vi "Parser.vi"(2 "error IO":errorcluster, 3 "ParserStateIN":T1) -> (0 "error out":errorcluster, 1 "ParserStateOUT":T1)   [LabVIEW 2010]
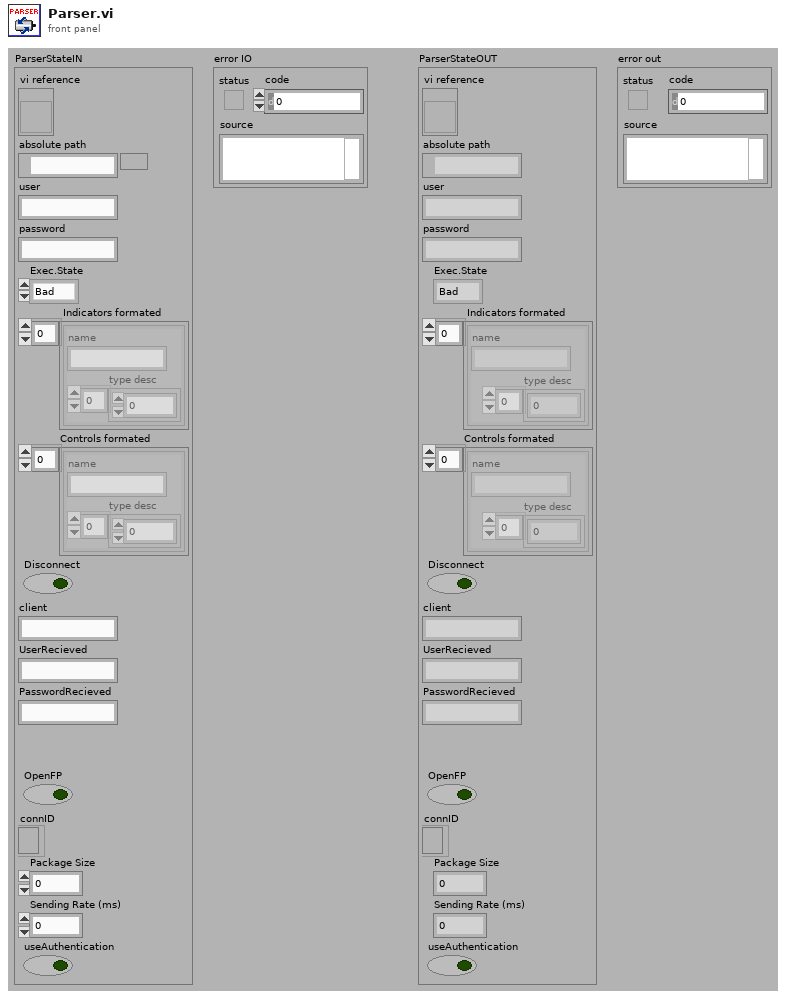
[diagram p1: front panel]
types:
  T1 = cluster{"vi reference":refnum<vi>, "absolute path":path, "user":string, "password":string, "Exec.State":enum32{"Bad", "Idle", "Run top level", "Running"}, " Indicators formated":cluster{"name":string, "type desc":i16[]}[], "Controls formated":cluster{"name":string, "type desc":i16[]}[], "Disconnect":bool, "client":string, "UserRecieved":string, "PasswordRecieved":string, "OpenFP":bool, "connID":refnum<k5>, "Package Size":u32, "Sending Rate (ms)":u32, "useAuthentication":bool}
  T2 = enum32{"Bad", "Idle", "Run top level", "Running"}
  T3 = enum16{"open", "replace", "create", "open or create", "replace or create", "replace or create with confirmation"}
  T4 = typedef "imagedata.ctl" = cluster{"image type":i32, "image depth":i32, "image":u8[], "mask":u8[], "colors":u32[], "Rectangle":cluster{"left":i16, "top":i16, "right":i16, "bottom":i16}}
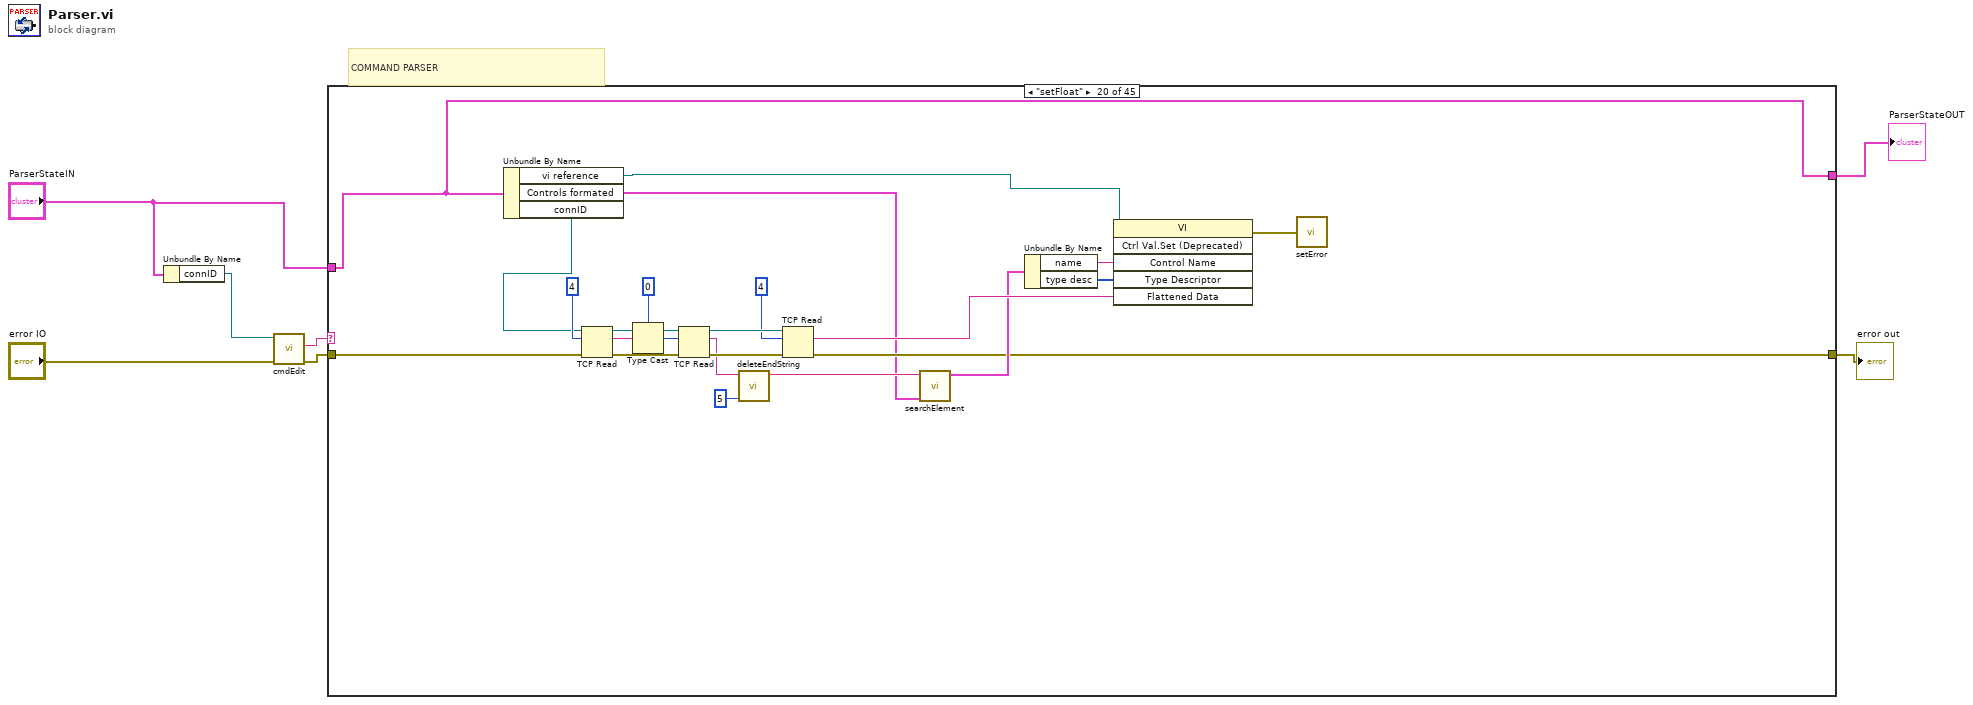
[diagram p0: block diagram]
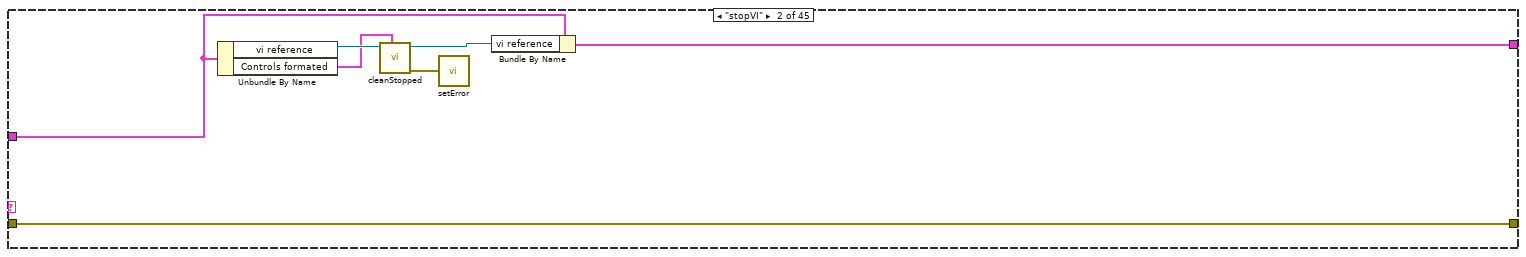
[diagram p3: hidden frame]
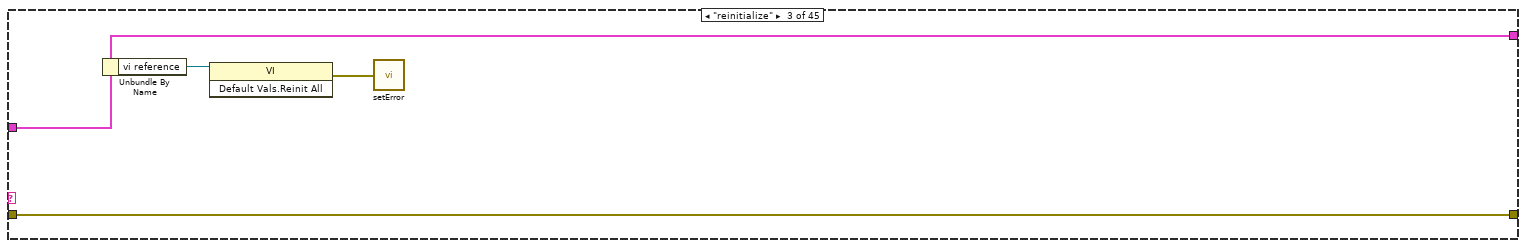
[diagram p4: hidden frame]
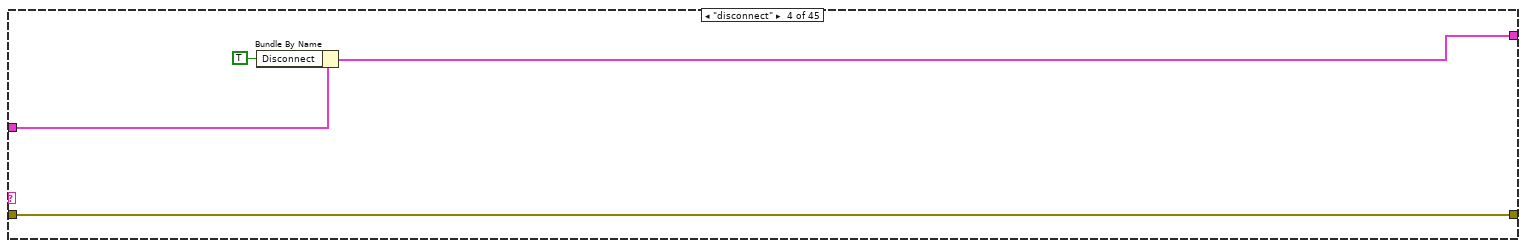
[diagram p5: hidden frame]
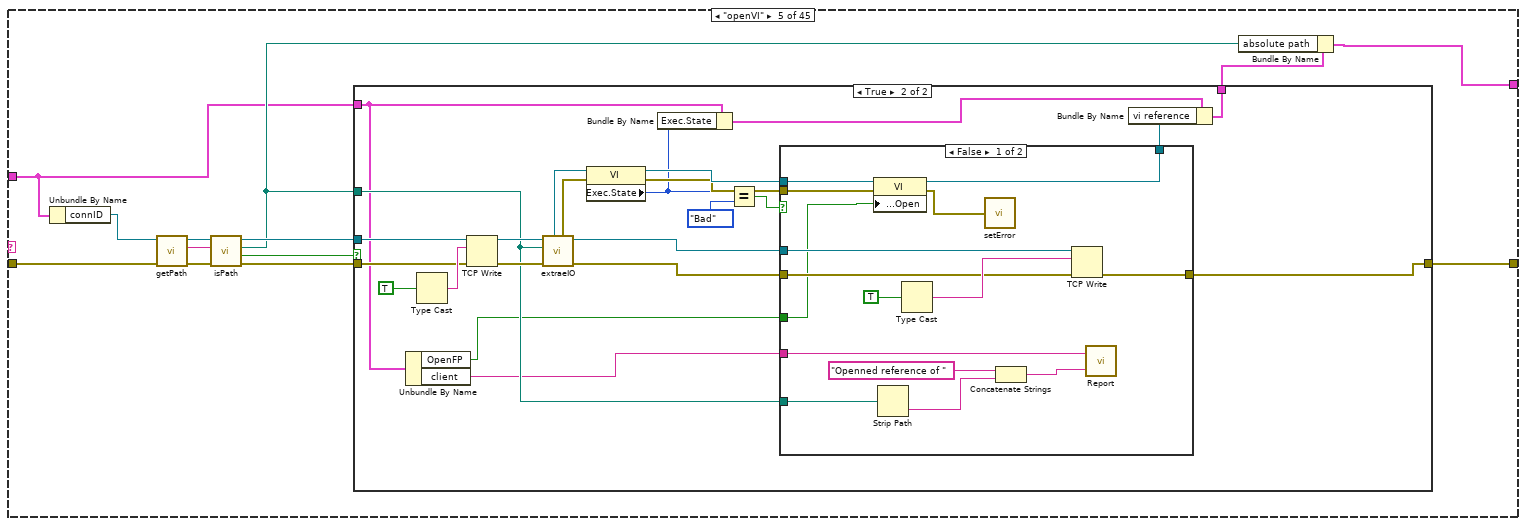
[diagram p6: hidden frame]
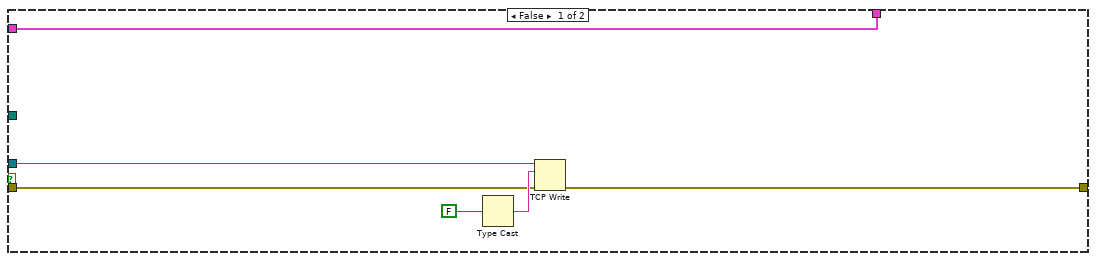
[diagram p7: hidden frame]
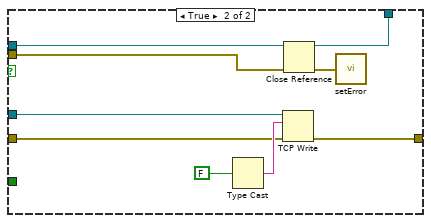
[diagram p8: hidden frame]
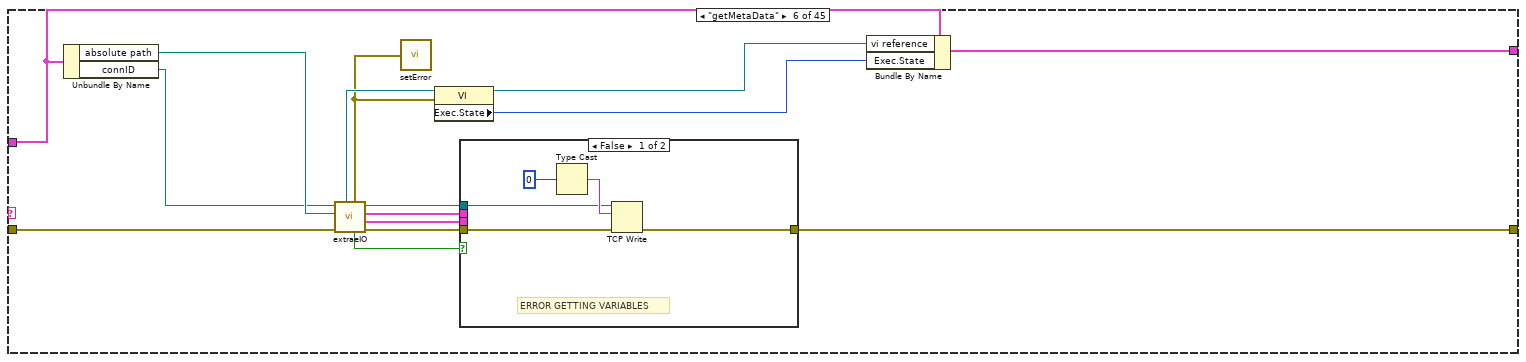
[diagram p9: hidden frame]
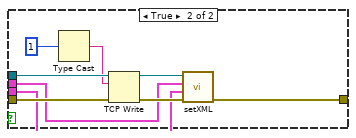
[diagram p10: hidden frame]
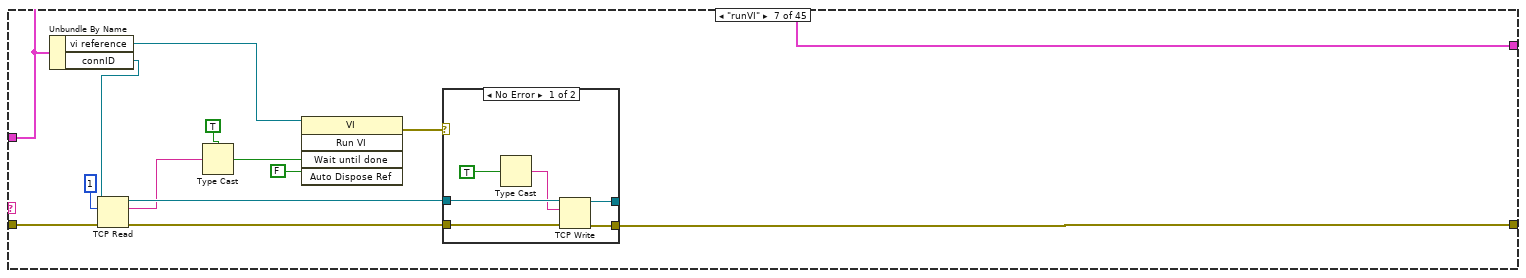
[diagram p11: hidden frame]
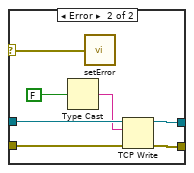
[diagram p12: hidden frame]
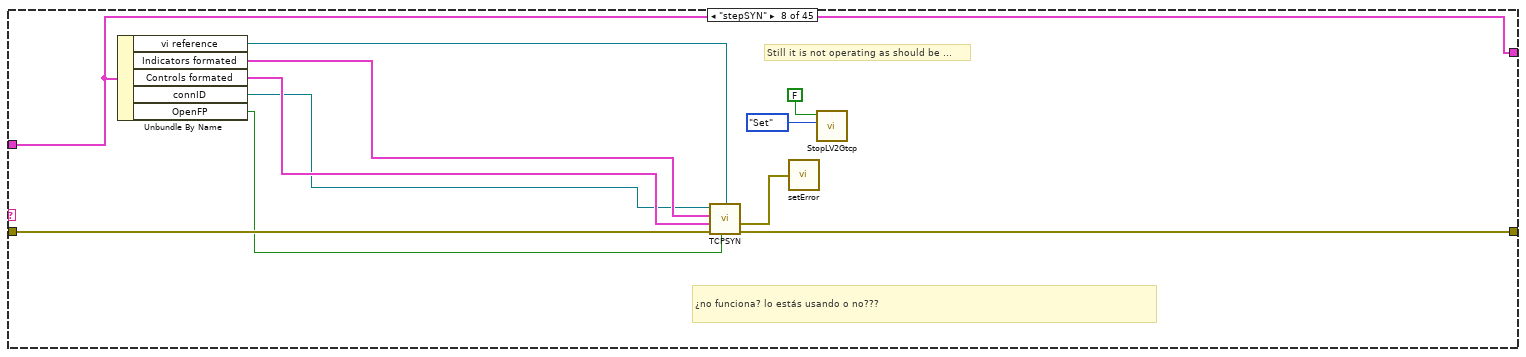
[diagram p13: hidden frame]
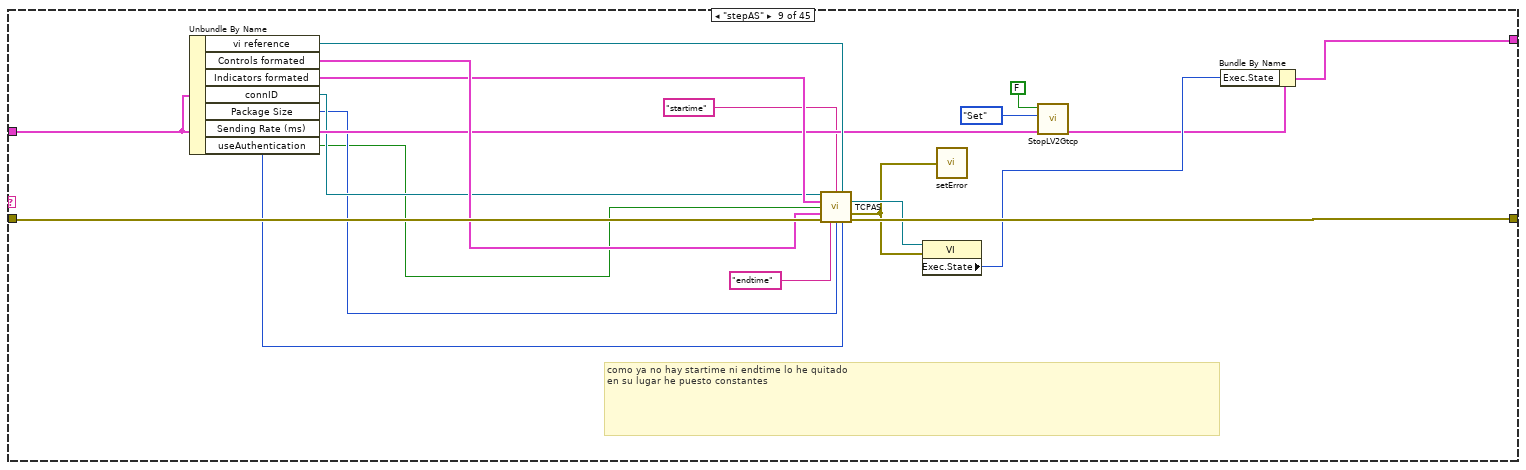
[diagram p14: hidden frame]
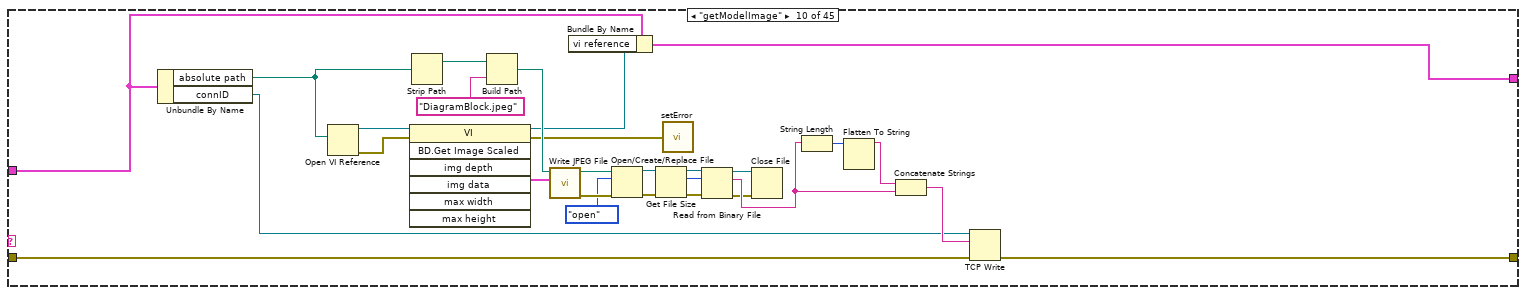
[diagram p15: hidden frame]
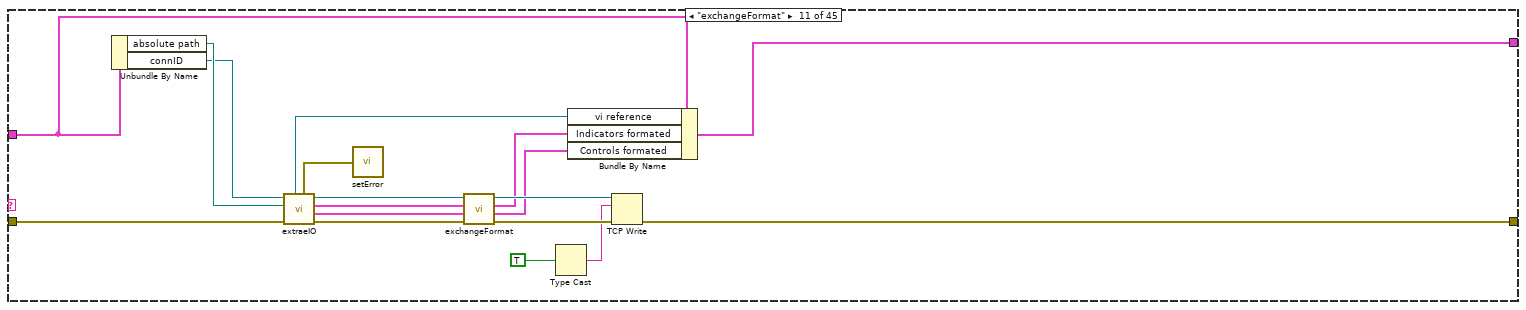
[diagram p16: hidden frame]
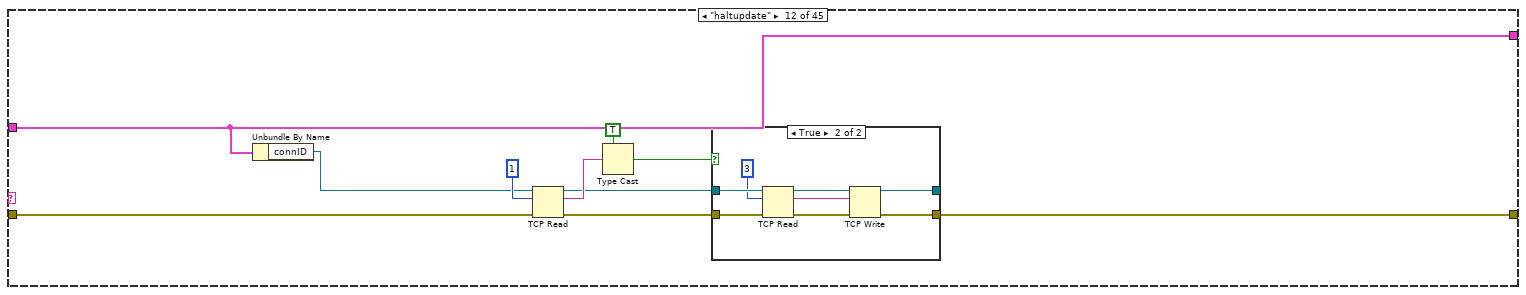
[diagram p17: hidden frame]
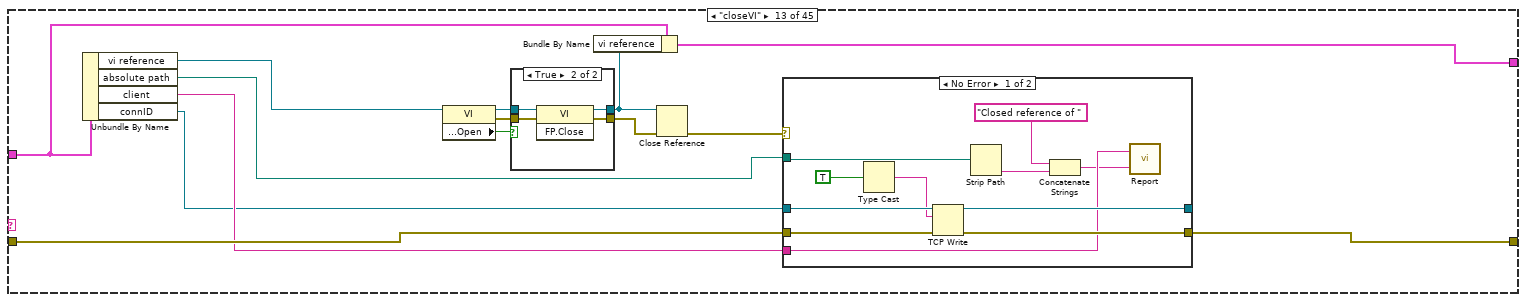
[diagram p19: hidden frame]
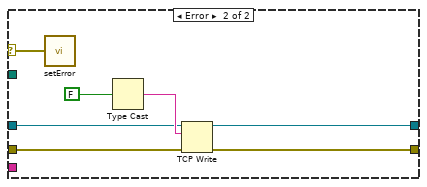
[diagram p20: hidden frame]
diagram:
  # "COMMAND PARSER"
  n1 = Unbundle By Name("ParserStateIN") -> ("connID"=w7:refnum<k5>)
  n2 = call "cmdEdit.vi"("error in (no error)"="error IO", "connection ID"=w7) -> ("error out"=w2:errorcluster, "Command"=w3:string)  [unwired: 8 out]
  n3 = case shown="\"setFloat\"" w3 {
    tunnel: w2 -> [w9 w16 w20 w24 w34 w100 w131 w155 w171 w197 w219 w229 w248 w296 w319 w326 w350 w372 w395 w424 w447 w478 w512 w549 w583 w618 w656 w694 w736 w780 w823 w841 w862 w883 w903 w925 w946 w967 w988 w1008 w1030 w1051 w1072 w1091 w1113]
    tunnel: [w9 w16 w20 w24 w30 w104 w129 w154 w170 w201 w212 w222 w247 w285 w319 w325 w349 w371 w394 w423 w446 w479 w511 w545 w584 w617 w655 w693 w731 w779 w819 w840 w861 w882 w902 w924 w945 w966 w987 w1007 w1029 w1050 w1071 w1092 w1112] -> w4
    tunnel: "ParserStateIN" -> [w8 w15 w17 w23 w26 w91 w120 w147 w163 w177 w206 w221 w245 w281 w318 w321 w344 w367 w390 w419 w442 w475 w508 w541 w580 w613 w651 w689 w727 w776 w816 w835 w856 w877 w900 w919 w942 w962 w982 w1003 w1026 w1045 w1066 w1087 w1109]
    tunnel: [w8 w10 w17 w21 w27 w92 w120 w147 w162 w175 w203 w221 w243 w284 w318 w321 w344 w367 w390 w419 w442 w475 w508 w541 w580 w613 w651 w689 w727 w776 w816 w835 w856 w877 w900 w919 w942 w962 w982 w1003 w1026 w1045 w1066 w1087 w1109] -> w5
    frame "", Default {
    }
    frame "stopVI" {
      n4 = Unbundle By Name(w15) -> ("vi reference"=w13:refnum<vi>, "Controls formated"=w11:cluster{"name":string, "type desc":i16[]}[])
      n5 = call "cleanStopped.vi"("input Controls"=w11, "vi reference in"=w13) -> ("error out"=w12:errorcluster, "vi reference out"=w14:refnum<vi>)  [unwired: 1 in, 7 out]
      n6 = call "setError.vi"("error"=w12) -> ()  [unwired: 1 out]
      n7 = Bundle By Name(cluster=w15, "vi reference"=w14) -> (w10:T1)
    }
    frame "reinitialize" {
      n8 = Unbundle By Name(w17) -> ("vi reference"=w18:refnum<vi>)
      n9 = invoke class="VI" method="Default Vals.Reinit All"(reference=w18) -> (error out=w19:errorcluster)  [unwired: 2 in, 2 out]
      n10 = call "setError.vi"("error"=w19) -> ()  [unwired: 1 out]
    }
    frame "disconnect" {
      n11 = Bundle By Name(cluster=w23, "Disconnect"=TRUE) -> (w21:T1)
    }
    frame "openVI" {
      n12 = Unbundle By Name(w26) -> ("connID"=w25:refnum<k5>)
      n13 = call "getPath.vi"("error in TCP"=w34, "connection ID in"=w25) -> ("error out TCP"=w35:errorcluster, "name vi"=w37:string, "connection ID out"=w36:refnum<k5>)  [unwired: 7 out]
      n14 = call "isPath.vi"("error in TCP"=w35, "string Path in"=w37, "connection ID in"=w36) -> ("error out TCP"=w32:errorcluster, "Path is Ok?"=w33:bool, "absolute path"=w28:path, "connection ID out"=w31:refnum<k5>)  [unwired: 1 in, 4 out]
      n15 = case shown="True" w33 {
        tunnel: w32 -> [w40 w63]
        tunnel: w31 -> [w41 w64]
        tunnel: [w39 w52] -> w30
        tunnel: w28 -> [_ w51]
        tunnel: w26 -> [w38 w46]
        tunnel: [w38 w47] -> w29
        frame False {
          n16 = Type Cast(x=FALSE) -> (*(type *) &x=w43:string)  [unwired: 1 out]
          n17 = TCP Write(connection ID=w41, data in=w43, error in (no error)=w40) -> (error out=w39:errorcluster)  [unwired: 3 out]
        }
        frame True {
          n18 = Unbundle By Name(w46) -> ("OpenFP"=w44:bool, "client"=w45:string)
          n19 = Type Cast(x=TRUE) -> (*(type *) &x=w66:string)  [unwired: 1 out]
          n20 = TCP Write(connection ID=w64, data in=w66, error in (no error)=w63) -> (connection ID out=w62:refnum<k5>, error out=w61:errorcluster)  [unwired: 2 out]
          n21 = call "extraeIO.vi"("error in TCP"=w61, "path"=w51, "connection IDin"=w62) -> ("error out TCP"=w53:errorcluster, "connection ID out"=w54:refnum<k5>, "error out"=w59:errorcluster, "vi reference"=w60:refnum<vi>)  [unwired: 5 out]
          n22 = property class="VI"(reference=w60, error in=w59) -> (reference out=w56:refnum<vi>, error out=w55:errorcluster, "Exec.State"=w50:T2)
          n23 = Bundle By Name(cluster=w46, "Exec.State"=w50) -> (w49:T1)
          n24 = Equal?(x=w50, y=T2."Bad") -> (x = y?=w58:bool)
          n25 = case shown="False" w58 {
            tunnel: w56 -> [w75 w82]
            tunnel: w55 -> [w74 w87]
            tunnel: w54 -> [w78 w86]
            tunnel: w53 -> [w77 w85]
            tunnel: [w76 w84] -> w52
            tunnel: w51 -> [w79 _]
            tunnel: [w73 w82] -> w48
            tunnel: w45 -> [w69 _]
            tunnel: w44 -> [w67 _]
            frame False {
              n26 = property class="VI"(reference=w75, error in=w74, "Front Panel.Open"=w67) -> (reference out=w73:refnum<vi>, error out=w72:errorcluster)
              n27 = Strip Path(path=w79) -> (name=w70:string)  [unwired: 1 out]
              n28 = Type Cast(x=TRUE) -> (*(type *) &x=w81:string)  [unwired: 1 out]
              n29 = call "setError.vi"("error"=w72) -> ()  [unwired: 1 out]
              n30 = Concatenate Strings("Openned reference of ", w70) -> (w68:string)
              n31 = TCP Write(connection ID=w78, data in=w81, error in (no error)=w77) -> (error out=w76:errorcluster)  [unwired: 3 out]
              n32 = call "Report.vi"("mesagge"=w68, "client"=w69) -> ()  [unwired: 1 in]
            }
            frame True {
              n33 = Type Cast(x=FALSE) -> (*(type *) &x=w89:string)  [unwired: 1 out]
              n34 = TCP Write(connection ID=w86, data in=w89, error in (no error)=w85) -> (error out=w84:errorcluster)  [unwired: 3 out]
              n35 = Close Reference(reference=w82, error in (no error)=w87) -> (error out=w83:errorcluster)
              n36 = call "setError.vi"("error"=w83) -> ()  [unwired: 1 out]
            }
          }
          n37 = Bundle By Name(cluster=w49, "vi reference"=w48) -> (w47:T1)
        }
      }
      n38 = Bundle By Name(cluster=w29, "absolute path"=w28) -> (w27:T1)
    }
    frame "getMetaData" {
      n39 = Unbundle By Name(w91) -> ("absolute path"=w95:path, "connID"=w90:refnum<k5>)
      n40 = call "extraeIO.vi"("error in TCP"=w100, "path"=w95, "connection IDin"=w90) -> ("error out TCP"=w102:errorcluster, "output Controls"=w98:cluster{"name":string, "type desc":i16[]}[], "output Indicators"=w103:cluster{"name":string, "type desc":i16[]}[], "connection ID out"=w101:refnum<k5>, "it is ok?"=w99:bool, "error out"=w96:errorcluster, "vi reference"=w97:refnum<vi>)  [unwired: 2 out]
      n41 = call "setError.vi"("error"=w96) -> ()  [unwired: 1 out]
      n42 = property class="VI"(reference=w97, error in=w96) -> (reference out=w94:refnum<vi>, "Exec.State"=w93:T2)  [unwired: 1 out]
      n43 = case shown="False" w99 {
        tunnel: w102 -> [w109 w116]
        tunnel: w103 -> [_ w111]
        tunnel: w98 -> [_ w110]
        tunnel: [w108 w118] -> w104
        tunnel: w101 -> [w105 w117]
        frame False {
          # "ERROR GETTING VARIABLES"
          n44 = Type Cast(x=0) -> (*(type *) &x=w107:string)  [unwired: 1 out]
          n45 = TCP Write(connection ID=w105, data in=w107, error in (no error)=w109) -> (error out=w108:errorcluster)  [unwired: 3 out]
        }
        frame True {
          n46 = Type Cast(x=1) -> (*(type *) &x=w112:string)  [unwired: 1 out]
          n47 = TCP Write(connection ID=w117, data in=w112, error in (no error)=w116) -> (connection ID out=w114:refnum<k5>, error out=w115:errorcluster)  [unwired: 2 out]
          n48 = call "setXML.vi"("error in"=w115, "Controls filtered"=w110, "Indicators filtered"=w111, "connection ID in"=w114) -> ("error out"=w118:errorcluster)  [unwired: 7 out]
        }
      }
      n49 = Bundle By Name(cluster=w91, "vi reference"=w94, "Exec.State"=w93) -> (w92:T1)
    }
    frame "runVI" {
      n50 = Unbundle By Name(w120) -> ("vi reference"=w121:refnum<vi>, "connID"=w119:refnum<k5>)
      n51 = TCP Read(connection ID=w119, bytes to read=1, error in (no error)=w131) -> (connection ID out=w128:refnum<k5>, data out=w123:string, error out=w127:errorcluster)  [unwired: 2 out]
      n52 = Type Cast(type=TRUE, x=w123) -> (*(type *) &x=w126:bool)
      n53 = invoke class="VI" method="Run VI"(reference=w121, "Wait until done"=w126, "Auto Dispose Ref"=FALSE ("Auto Dispose Reference")) -> (error out=w130:errorcluster)  [unwired: 2 in, 4 out]
      n54 = case shown="No Error" w130 {
        selector: w130 -> [_ w138]
        tunnel: w128 -> [w137 w144]
        tunnel: w127 -> [w136 w143]
        tunnel: [w135 w142] -> _
        tunnel: [w134 w141] -> w129
        frame No Error {
          n55 = Type Cast(x=TRUE) -> (*(type *) &x=w132:string)  [unwired: 1 out]
          n56 = TCP Write(connection ID=w137, data in=w132, error in (no error)=w136) -> (connection ID out=w135:refnum<k5>, error out=w134:errorcluster)  [unwired: 2 out]
        }
        frame Error {
          n57 = Type Cast(x=FALSE) -> (*(type *) &x=w139:string)  [unwired: 1 out]
          n58 = call "setError.vi"("error"=w138) -> ()  [unwired: 1 out]
          n59 = TCP Write(connection ID=w144, data in=w139, error in (no error)=w143) -> (connection ID out=w142:refnum<k5>, error out=w141:errorcluster)  [unwired: 2 out]
        }
      }
    }
    frame "stepSYN" {
      # "¿no funciona? lo estás usando o no???"
      # "Still it is not operating as should be ..."
      n60 = Unbundle By Name(w147) -> ("vi reference"=w150:refnum<vi>, "Indicators formated"=w149:cluster{"name":string, "type desc":i16[]}[], "Controls formated"=w148:cluster{"name":string, "type desc":i16[]}[], "connID"=w146:refnum<k5>, "OpenFP"=w145:bool)
      n61 = call "TCPSYN.vi"("vi reference"=w150, "Front Panel Window:Open"=w145, "error in TCP"=w155, "input Controls"=w148, "input Indicators"=w149, "connection ID in"=w146) -> ("error TCP out"=w154:errorcluster, "error out"=w151:errorcluster)  [unwired: 1 in, 3 out]
      n62 = call "setError.vi"("error"=w151) -> ()  [unwired: 1 out]
      n63 = call "StopLV2Gtcp.vi"("Mode"=enum16{"Init", "Get", "Set"}."Set", "Stop IN"=FALSE) -> ()  [unwired: 10 out]
    }
    frame "stepAS" {
      # "como ya no hay startime ni endtime lo he quitado\nen su lugar he puesto constantes"
      n64 = Unbundle By Name(w163) -> ("vi reference"=w167:refnum<vi>, "Controls formated"=w166:cluster{"name":string, "type desc":i16[]}[], "Indicators formated"=w165:cluster{"name":string, "type desc":i16[]}[], "connID"=w159:refnum<k5>, "Package Size"=w158:u32, "Sending Rate (ms)"=w157:u32, "useAuthentication"=w156:bool)
      n65 = call "TCPAS.vi"("connection ID in"=w159, "starttime"="startime", "vi reference"=w167, "input Indicators"=w165, "rejectbyendtime"=w156, "input Controls"=w166, "error in TCP"=w171, "endtime"="endtime", "packageSize"=w158, "Sent rate (ms)"=w157) -> ("vi reference"=w169:refnum<vi>, "error out"=w168:errorcluster, "error TCP out"=w170:errorcluster)  [unwired: 1 in, 2 out]
      n66 = property class="VI"(reference=w169, error in=w168) -> ("Exec.State"=w164:T2)  [unwired: 2 out]
      n67 = call "setError.vi"("error"=w168) -> ()  [unwired: 1 out]
      n68 = call "StopLV2Gtcp.vi"("Mode"=enum16{"Init", "Get", "Set"}."Set", "Stop IN"=FALSE) -> ()  [unwired: 10 out]
      n69 = Bundle By Name(cluster=w163, "Exec.State"=w164) -> (w162:T1)
    }
    frame "getModelImage" {
      n70 = Unbundle By Name(w177) -> ("absolute path"=w178:path, "connID"=w174:refnum<k5>)
      n71 = Open VI Reference(vi path=w178) -> (vi reference=w196:refnum<vi>, error out=w195:errorcluster)  [unwired: 1 in, 4 out]
      n72 = invoke class="VI" method="BD.Get Image Scaled"(reference=w196, error in=w195) -> (reference out=w176:refnum<vi>, error out=w179:errorcluster, "img data"=w194:T4)  [unwired: 5 in, 4 out]
      n73 = Strip Path(path=w178) -> (stripped path=w200:path)  [unwired: 1 out]
      n74 = Build Path(base path=w200, name or relative path="DiagramBlock.jpeg") -> (appended path=w198:path)
      n75 = call <vilib>:"Write JPEG File.vi"("image data"=w194, "path to JPEG file"=w198) -> ("error out"=w187:errorcluster, "path"=w188:path)  [unwired: 1 in, 7 out]
      n76 = Bundle By Name(cluster=w177, "vi reference"=w176) -> (w175:T1)
      n77 = Open/Create/Replace File(file path (use dialog)=w188, error in=w187, operation (0:open)=T3."open") -> (refnum out=w189:refnum<file>, error out=w190:errorcluster)  [unwired: 3 in, 1 out]
      n78 = Get File Size(file=w189, error in=w190) -> (refnum out=w185:refnum<file>, size (in bytes)=w184:i64, 0:w183:errorcluster)
      n79 = call "setError.vi"("error"=w179) -> ()  [unwired: 1 out]
      n80 = Read from Binary File(8:w183, 10:w184, 11:w185) -> (0:w181:errorcluster, 2:w193:string, 3:w182:refnum<file>)  [unwired: 4 out]
      n81 = Close File(refnum=w182, error in=w181) -> ()  [unwired: 2 out]
      n82 = String Length(string=w193) -> (length=w180:i32)
      n83 = Flatten To String(anything=w180) -> (data string=w192:string)  [unwired: 1 in, 4 out]
      n84 = Concatenate Strings(w192, w193) -> (w191:string)
      n85 = TCP Write(connection ID=w174, data in=w191, error in (no error)=w197) -> (error out=w201:errorcluster)  [unwired: 3 out]
    }
    frame "exchangeFormat" {
      n86 = Unbundle By Name(w206) -> ("absolute path"=w208:path, "connID"=w202:refnum<k5>)
      n87 = call "extraeIO.vi"("error in TCP"=w219, "path"=w208, "connection IDin"=w202) -> ("error out TCP"=w217:errorcluster, "output Controls"=w215:cluster{"name":string, "type desc":i16[]}[], "output Indicators"=w216:cluster{"name":string, "type desc":i16[]}[], "connection ID out"=w218:refnum<k5>, "error out"=w209:errorcluster, "vi reference"=w207:refnum<vi>)  [unwired: 3 out]
      n88 = call "setError.vi"("error"=w209) -> ()  [unwired: 1 out]
      n89 = call "exchangeFormat.vi"("error in TCP"=w217, "input Controls"=w215, "input Indicators"=w216, "connection ID in"=w218) -> ("error out TCP"=w213:errorcluster, "output Controls"=w204:cluster{"name":string, "type desc":i16[]}[], "output Indicators"=w205:cluster{"name":string, "type desc":i16[]}[], "connection ID out"=w214:refnum<k5>)  [unwired: 4 out]
      n90 = Type Cast(x=TRUE) -> (*(type *) &x=w211:string)  [unwired: 1 out]
      n91 = Bundle By Name(cluster=w206, "vi reference"=w207, "Indicators formated"=w205, "Controls formated"=w204) -> (w203:T1)
      n92 = TCP Write(connection ID=w214, data in=w211, error in (no error)=w213) -> (error out=w212:errorcluster)  [unwired: 3 out]
    }
    frame "haltupdate" {
      n93 = Unbundle By Name(w221) -> ("connID"=w220:refnum<k5>)
      n94 = TCP Read(connection ID=w220, bytes to read=1, error in (no error)=w229) -> (connection ID out=w224:refnum<k5>, data out=w227:string, error out=w223:errorcluster)  [unwired: 2 out]
      n95 = Type Cast(type=TRUE, x=w227) -> (*(type *) &x=w225:bool)
      n96 = case shown="True" w225 {
        tunnel: w224 -> [w231 w239]
        tunnel: w223 -> [w230 w238]
        tunnel: [w231 w233] -> _
        tunnel: [w230 w232] -> w222
        frame False {
        }
        frame True {
          n97 = TCP Read(connection ID=w239, bytes to read=3, error in (no error)=w238) -> (connection ID out=w237:refnum<k5>, data out=w235:string, error out=w236:errorcluster)  [unwired: 2 out]
          n98 = TCP Write(connection ID=w237, data in=w235, error in (no error)=w236) -> (connection ID out=w233:refnum<k5>, error out=w232:errorcluster)  [unwired: 2 out]
        }
      }
    }
    frame "closeVI" {
      n99 = Unbundle By Name(w245) -> ("vi reference"=w246:refnum<vi>, "absolute path"=w242:path, "client"=w241:string, "connID"=w240:refnum<k5>)
      n100 = property class="VI"(reference=w246) -> (reference out=w251:refnum<vi>, error out=w252:errorcluster, "Front Panel.Open"=w253:bool)  [unwired: 1 in]
      n101 = case shown="True" w253 {
        tunnel: w251 -> [w273 w277]
        tunnel: w252 -> [w272 w274]
        tunnel: [w273 w276] -> w244
        tunnel: [w272 w275] -> w250
        frame False {
        }
        frame True {
          n102 = invoke class="VI" method="FP.Close"(reference=w277, error in=w274) -> (reference out=w276:refnum<vi>, error out=w275:errorcluster)  [unwired: 1 in, 1 out]
        }
      }
      n103 = Bundle By Name(cluster=w245, "vi reference"=w244) -> (w243:T1)
      n104 = Close Reference(reference=w244, error in (no error)=w250) -> (error out=w249:errorcluster)
      n105 = case shown="No Error" w249 {
        selector: w249 -> [_ w265]
        tunnel: w240 -> [w263 w269]
        tunnel: w248 -> [w264 w268]
        tunnel: [w260 w267] -> _
        tunnel: [w259 w266] -> w247
        tunnel: w242 -> [w258 _]
        tunnel: w241 -> [w257 _]
        frame No Error {
          n106 = Type Cast(x=TRUE) -> (*(type *) &x=w261:string)  [unwired: 1 out]
          n107 = TCP Write(connection ID=w263, data in=w261, error in (no error)=w264) -> (connection ID out=w260:refnum<k5>, error out=w259:errorcluster)  [unwired: 2 out]
          n108 = Strip Path(path=w258) -> (name=w255:string)  [unwired: 1 out]
          n109 = Concatenate Strings("Closed reference of " ("string"), w255) -> (w256:string)
          n110 = call "Report.vi"("mesagge"=w256, "client"=w257) -> ()  [unwired: 1 in]
        }
        frame Error {
          n111 = call "setError.vi"("error"=w265) -> ()  [unwired: 1 out]
          n112 = Type Cast(x=FALSE) -> (*(type *) &x=w270:string)  [unwired: 1 out]
          n113 = TCP Write(connection ID=w269, data in=w270, error in (no error)=w268) -> (connection ID out=w267:refnum<k5>, error out=w266:errorcluster)  [unwired: 2 out]
        }
      }
    }
    frame "authenticate" {
      # "Esto habría que cambiarlo un poco"
      # "Timeleft ya no es útil\ndevuelve constantes"
      n114 = Unbundle By Name(w281) -> ("user"=w280:string, "password"=w279:string, "connID"=w278:refnum<k5>)
      n115 = call "userpassReceptor.vi"("error in (no error)"=w296, "connection ID"=w278) -> ("error out"=w294:errorcluster, "password"=w282:string, "user"=w283:string, "connection ID out"=w295:refnum<k5>)  [unwired: 2 out]
      n116 = Bundle By Name(cluster=w281, "UserRecieved"=w283, "PasswordRecieved"=w282) -> (w284:T1)
      n117 = call "CheckUserPass.vi"("password"=w279, "user"=w280, "error in"=w294, "PasswordRecieved"=w282, "UserRecieved"=w283, "connection ID in"=w295) -> ("error out"=w298:errorcluster, "connection ID out"=w297:refnum<k5>, "result"=w299:bool)  [unwired: 3 out]
      n118 = case shown="False" w299 {
        tunnel: [w312 w317] -> w290
        tunnel: w298 -> [w313 w315]
        tunnel: w297 -> [w314 w316]
        tunnel: [w314 w316] -> w293
        tunnel: [w313 w315] -> w292
        frame False {
          w312 = 0 items=["user and pass no exist", "no match with timeslot", "user ok"] ("result")
        }
        frame True {
          w317 = 2 items=["user and pass no exist", "no match with timeslot", "user ok"] ("result")
        }
      }
      n119 = Type Cast(x=w290) -> (*(type *) &x=w291:string)  [unwired: 1 out]
      n120 = TCP Write(connection ID=w293, data in=w291, error in (no error)=w292) -> (connection ID out=w287:refnum<k5>, error out=w286:errorcluster)  [unwired: 2 out]
      n121 = Equal?(x=w290, y=2) -> (x = y?=w288:bool)
      n122 = case shown="True" w288 {
        tunnel: w287 -> [w301 w311]
        tunnel: w286 -> [w300 w310]
        tunnel: [w301 w307] -> _
        tunnel: [w300 w306] -> w285
        frame False {
        }
        frame True {
          n123 = Type Cast(x=ext 0.0) -> (*(type *) &x=w305:string)  [unwired: 1 out]
          n124 = Type Cast(x=ext 0.0) -> (*(type *) &x=w304:string)  [unwired: 1 out]
          n125 = TCP Write(connection ID=w311, data in=w305, error in (no error)=w310) -> (connection ID out=w308:refnum<k5>, error out=w309:errorcluster)  [unwired: 2 out]
          n126 = TCP Write(connection ID=w308, data in=w304, error in (no error)=w309) -> (connection ID out=w307:refnum<k5>, error out=w306:errorcluster)  [unwired: 2 out]
        }
      }
    }
    frame "clientKeepAlive" {
    }
    frame "setBoolean" {
      n127 = Unbundle By Name(w321) -> ("vi reference"=w323:refnum<vi>, "Controls formated"=w322:cluster{"name":string, "type desc":i16[]}[], "connID"=w320:refnum<k5>)
      n128 = TCP Read(connection ID=w320, bytes to read=4, error in (no error)=w326) -> (connection ID out=w335:refnum<k5>, data out=w338:string, error out=w334:errorcluster)  [unwired: 2 out]
      n129 = Type Cast(type=0, x=w338) -> (*(type *) &x=w336:i32)
      n130 = TCP Read(connection ID=w335, bytes to read=w336, error in (no error)=w334) -> (connection ID out=w332:refnum<k5>, data out=w329:string, error out=w333:errorcluster)  [unwired: 2 out]
      n131 = TCP Read(connection ID=w332, bytes to read=1, error in (no error)=w333) -> (data out=w330:string, error out=w325:errorcluster)  [unwired: 3 out]
      n132 = call "deleteEndString.vi"("chars to delete"=5, "string in"=w329) -> ("substring out"=w328:string)  [unwired: 9 out]
      n133 = call "searchElement.vi"("input"=w322, "name"=w328) -> ("output"=w341:cluster{"name":string, "type desc":i16[]})  [unwired: 9 out]
      n134 = Unbundle By Name(w341) -> ("name"=w340:string, "type desc"=w339:i16[])
      n135 = invoke class="VI" method="Ctrl Val.Set (Deprecated)"(reference=w323, "Control Name"=w340, "Type Descriptor"=w339, "Flattened Data"=w330) -> (error out=w324:errorcluster)  [unwired: 2 in, 5 out]
      n136 = call "setError.vi"("error"=w324) -> ()  [unwired: 1 out]
    }
    frame "setInt" {
      n137 = Unbundle By Name(w344) -> ("vi reference"=w346:refnum<vi>, "Controls formated"=w345:cluster{"name":string, "type desc":i16[]}[], "connID"=w343:refnum<k5>)
      n138 = TCP Read(connection ID=w343, bytes to read=4, error in (no error)=w350) -> (connection ID out=w362:refnum<k5>, data out=w361:string, error out=w364:errorcluster)  [unwired: 2 out]
      n139 = Type Cast(type=0, x=w361) -> (*(type *) &x=w360:i32)
      n140 = TCP Read(connection ID=w362, bytes to read=w360, error in (no error)=w364) -> (connection ID out=w359:refnum<k5>, data out=w356:string, error out=w358:errorcluster)  [unwired: 2 out]
      n141 = call "deleteEndString.vi"("chars to delete"=5 ("y"), "string in"=w356) -> ("substring out"=w351:string)  [unwired: 9 out]
      n142 = TCP Read(connection ID=w359, bytes to read=4, error in (no error)=w358) -> (data out=w352:string, error out=w349:errorcluster)  [unwired: 3 out]
      n143 = call "searchElement.vi"("input"=w345, "name"=w351) -> ("output"=w355:cluster{"name":string, "type desc":i16[]})  [unwired: 9 out]
      n144 = Unbundle By Name(w355) -> ("name"=w354:string, "type desc"=w353:i16[])
      n145 = invoke class="VI" method="Ctrl Val.Set (Deprecated)"(reference=w346, "Control Name"=w354, "Type Descriptor"=w353, "Flattened Data"=w352) -> (error out=w347:errorcluster)  [unwired: 2 in, 5 out]
      n146 = call "setError.vi"("error"=w347) -> ()  [unwired: 1 out]
    }
    frame "setDouble" {
      n147 = Unbundle By Name(w367) -> ("vi reference"=w369:refnum<vi>, "Controls formated"=w368:cluster{"name":string, "type desc":i16[]}[], "connID"=w366:refnum<k5>)
      n148 = TCP Read(connection ID=w366, bytes to read=4, error in (no error)=w372) -> (connection ID out=w385:refnum<k5>, data out=w384:string, error out=w387:errorcluster)  [unwired: 2 out]
      n149 = Type Cast(type=0, x=w384) -> (*(type *) &x=w383:i32)
      n150 = TCP Read(connection ID=w385, bytes to read=w383, error in (no error)=w387) -> (connection ID out=w382:refnum<k5>, data out=w374:string, error out=w381:errorcluster)  [unwired: 2 out]
      n151 = call "deleteEndString.vi"("chars to delete"=5 ("y"), "string in"=w374) -> ("substring out"=w373:string)  [unwired: 9 out]
      n152 = TCP Read(connection ID=w382, bytes to read=8, error in (no error)=w381) -> (data out=w380:string, error out=w371:errorcluster)  [unwired: 3 out]
      n153 = call "searchElement.vi"("input"=w368, "name"=w373) -> ("output"=w379:cluster{"name":string, "type desc":i16[]})  [unwired: 9 out]
      n154 = Unbundle By Name(w379) -> ("name"=w378:string, "type desc"=w377:i16[])
      n155 = invoke class="VI" method="Ctrl Val.Set (Deprecated)"(reference=w369, "Control Name"=w378, "Type Descriptor"=w377, "Flattened Data"=w380) -> (error out=w370:errorcluster)  [unwired: 2 in, 5 out]
      n156 = call "setError.vi"("error"=w370) -> ()  [unwired: 1 out]
    }
    frame "setString" {
      n157 = Unbundle By Name(w390) -> ("vi reference"=w392:refnum<vi>, "Controls formated"=w391:cluster{"name":string, "type desc":i16[]}[], "connID"=w389:refnum<k5>)
      n158 = TCP Read(connection ID=w389, bytes to read=4, error in (no error)=w395) -> (connection ID out=w414:refnum<k5>, data out=w413:string, error out=w416:errorcluster)  [unwired: 2 out]
      n159 = Type Cast(type=0, x=w413) -> (*(type *) &x=w412:i32)
      n160 = TCP Read(connection ID=w414, bytes to read=w412, error in (no error)=w416) -> (connection ID out=w411:refnum<k5>, data out=w400:string, error out=w410:errorcluster)  [unwired: 2 out]
      n161 = call "deleteEndString.vi"("chars to delete"=5, "string in"=w400) -> ("substring out"=w398:string)  [unwired: 9 out]
      n162 = TCP Read(connection ID=w411, bytes to read=4, error in (no error)=w410) -> (connection ID out=w404:refnum<k5>, data out=w402:string, error out=w405:errorcluster)  [unwired: 2 out]
      n163 = Type Cast(type=0, x=w402) -> (*(type *) &x=w401:i32)
      n164 = call "searchElement.vi"("input"=w391, "name"=w398) -> ("output"=w409:cluster{"name":string, "type desc":i16[]})  [unwired: 9 out]
      n165 = TCP Read(connection ID=w404, bytes to read=w401, error in (no error)=w405) -> (data out=w397:string, error out=w394:errorcluster)  [unwired: 3 out]
      n166 = Variant To Flattened String(Variant=w397) -> (data string=w396:string)  [unwired: 1 out]
      n167 = Unbundle By Name(w409) -> ("name"=w408:string, "type desc"=w407:i16[])
      n168 = invoke class="VI" method="Ctrl Val.Set (Deprecated)"(reference=w392, "Control Name"=w408, "Type Descriptor"=w407, "Flattened Data"=w396) -> (error out=w393:errorcluster)  [unwired: 2 in, 5 out]
      n169 = call "setError.vi"("error"=w393) -> ()  [unwired: 1 out]
    }
    frame "setFloat" {
      n170 = Unbundle By Name(w419) -> ("vi reference"=w421:refnum<vi>, "Controls formated"=w420:cluster{"name":string, "type desc":i16[]}[], "connID"=w418:refnum<k5>)
      n171 = TCP Read(connection ID=w418, bytes to read=4, error in (no error)=w424) -> (connection ID out=w437:refnum<k5>, data out=w436:string, error out=w439:errorcluster)  [unwired: 2 out]
      n172 = Type Cast(type=0, x=w436) -> (*(type *) &x=w435:i32)
      n173 = TCP Read(connection ID=w437, bytes to read=w435, error in (no error)=w439) -> (connection ID out=w434:refnum<k5>, data out=w426:string, error out=w433:errorcluster)  [unwired: 2 out]
      n174 = call "deleteEndString.vi"("chars to delete"=5 ("y"), "string in"=w426) -> ("substring out"=w425:string)  [unwired: 9 out]
      n175 = TCP Read(connection ID=w434, bytes to read=4, error in (no error)=w433) -> (data out=w432:string, error out=w423:errorcluster)  [unwired: 3 out]
      n176 = call "searchElement.vi"("input"=w420, "name"=w425) -> ("output"=w431:cluster{"name":string, "type desc":i16[]})  [unwired: 9 out]
      n177 = Unbundle By Name(w431) -> ("name"=w430:string, "type desc"=w429:i16[])
      n178 = invoke class="VI" method="Ctrl Val.Set (Deprecated)"(reference=w421, "Control Name"=w430, "Type Descriptor"=w429, "Flattened Data"=w432) -> (error out=w422:errorcluster)  [unwired: 2 in, 5 out]
      n179 = call "setError.vi"("error"=w422) -> ()  [unwired: 1 out]
    }
    frame "setBooleanArray" {
      n180 = Unbundle By Name(w442) -> ("connID"=w441:refnum<k5>, "vi reference"=w444:refnum<vi>, "Controls formated"=w443:cluster{"name":string, "type desc":i16[]}[])
      n181 = TCP Read(connection ID=w441, bytes to read=4, error in (no error)=w447) -> (connection ID out=w471:refnum<k5>, data out=w470:string, error out=w473:errorcluster)  [unwired: 2 out]
      n182 = Type Cast(type=0, x=w470) -> (*(type *) &x=w469:i32)
      n183 = TCP Read(connection ID=w471, bytes to read=w469, error in (no error)=w473) -> (connection ID out=w468:refnum<k5>, data out=w460:string, error out=w467:errorcluster)  [unwired: 2 out]
      n184 = call "deleteEndString.vi"("chars to delete"=5 ("y"), "string in"=w460) -> ("substring out"=w461:string)  [unwired: 9 out]
      n185 = TCP Read(connection ID=w468, bytes to read=4, error in (no error)=w467) -> (connection ID out=w465:refnum<k5>, data out=w463:string, error out=w466:errorcluster)  [unwired: 2 out]
      n186 = Type Cast(type=0, x=w463) -> (*(type *) &x=w454:i32)
      n187 = Multiply(x=1, y=w454) -> (x*y=w456:i32)
      n188 = call "searchElement.vi"("input"=w443, "name"=w461) -> ("output"=w457:cluster{"name":string, "type desc":i16[]})  [unwired: 9 out]
      n189 = TCP Read(connection ID=w465, bytes to read=w456, error in (no error)=w466) -> (data out=w452:string, error out=w446:errorcluster)  [unwired: 3 out]
      n190 = Unflatten From String(type=bool[] [], binary string=w452, data includes array or string size? (T)=FALSE) -> (value=w450:bool[])  [unwired: 1 in, 3 out]
      n191 = Variant To Flattened String(Variant=w450) -> (data string=w453:string)  [unwired: 1 out]
      n192 = Unbundle By Name(w457) -> ("name"=w459:string, "type desc"=w458:i16[])
      n193 = invoke class="VI" method="Ctrl Val.Set (Deprecated)"(reference=w444, "Control Name"=w459, "Type Descriptor"=w458, "Flattened Data"=w453) -> ()  [unwired: 2 in, 6 out]
    }
    frame "setIntArray" {
      n194 = Unbundle By Name(w475) -> ("vi reference"=w477:refnum<vi>, "Controls formated"=w476:cluster{"name":string, "type desc":i16[]}[], "connID"=w474:refnum<k5>)
      n195 = TCP Read(connection ID=w474, bytes to read=4, error in (no error)=w478) -> (connection ID out=w504:refnum<k5>, data out=w503:string, error out=w506:errorcluster)  [unwired: 2 out]
      n196 = Type Cast(type=0, x=w503) -> (*(type *) &x=w502:i32)
      n197 = TCP Read(connection ID=w504, bytes to read=w502, error in (no error)=w506) -> (connection ID out=w501:refnum<k5>, data out=w493:string, error out=w500:errorcluster)  [unwired: 2 out]
      n198 = call "deleteEndString.vi"("chars to delete"=5 ("y"), "string in"=w493) -> ("substring out"=w494:string)  [unwired: 9 out]
      n199 = TCP Read(connection ID=w501, bytes to read=4, error in (no error)=w500) -> (connection ID out=w498:refnum<k5>, data out=w496:string, error out=w499:errorcluster)  [unwired: 2 out]
      n200 = Type Cast(type=0, x=w496) -> (*(type *) &x=w487:i32)
      n201 = Multiply(x=4, y=w487) -> (x*y=w489:i32)
      n202 = call "searchElement.vi"("input"=w476, "name"=w494) -> ("output"=w490:cluster{"name":string, "type desc":i16[]})  [unwired: 9 out]
      n203 = TCP Read(connection ID=w498, bytes to read=w489, error in (no error)=w499) -> (data out=w485:string, error out=w479:errorcluster)  [unwired: 3 out]
      n204 = Unflatten From String(type=i32[] [], binary string=w485, data includes array or string size? (T)=FALSE) -> (value=w482:i32[])  [unwired: 1 in, 3 out]
      n205 = Variant To Flattened String(Variant=w482) -> (data string=w486:string)  [unwired: 1 out]
      n206 = Unbundle By Name(w490) -> ("name"=w492:string, "type desc"=w491:i16[])
      n207 = invoke class="VI" method="Ctrl Val.Set (Deprecated)"(reference=w477, "Control Name"=w492, "Type Descriptor"=w491, "Flattened Data"=w486) -> ()  [unwired: 2 in, 6 out]
    }
    frame "setDoubleArray" {
      n208 = Unbundle By Name(w508) -> ("vi reference"=w510:refnum<vi>, "Controls formated"=w509:cluster{"name":string, "type desc":i16[]}[], "connID"=w507:refnum<k5>)
      n209 = TCP Read(connection ID=w507, bytes to read=4, error in (no error)=w512) -> (connection ID out=w537:refnum<k5>, data out=w536:string, error out=w539:errorcluster)  [unwired: 2 out]
      n210 = Type Cast(type=0, x=w536) -> (*(type *) &x=w535:i32)
      n211 = TCP Read(connection ID=w537, bytes to read=w535, error in (no error)=w539) -> (connection ID out=w534:refnum<k5>, data out=w526:string, error out=w533:errorcluster)  [unwired: 2 out]
      n212 = call "deleteEndString.vi"("chars to delete"=5 ("y"), "string in"=w526) -> ("substring out"=w527:string)  [unwired: 9 out]
      n213 = TCP Read(connection ID=w534, bytes to read=4, error in (no error)=w533) -> (connection ID out=w531:refnum<k5>, data out=w529:string, error out=w532:errorcluster)  [unwired: 2 out]
      n214 = Type Cast(type=0, x=w529) -> (*(type *) &x=w520:i32)
      n215 = Multiply(x=8, y=w520) -> (x*y=w522:i32)
      n216 = call "searchElement.vi"("input"=w509, "name"=w527) -> ("output"=w523:cluster{"name":string, "type desc":i16[]})  [unwired: 9 out]
      n217 = TCP Read(connection ID=w531, bytes to read=w522, error in (no error)=w532) -> (data out=w518:string, error out=w511:errorcluster)  [unwired: 3 out]
      n218 = Unflatten From String(type=dbl[] [], binary string=w518, data includes array or string size? (T)=FALSE) -> (value=w515:dbl[])  [unwired: 1 in, 3 out]
      n219 = Variant To Flattened String(Variant=w515) -> (data string=w519:string)  [unwired: 1 out]
      n220 = Unbundle By Name(w523) -> ("name"=w525:string, "type desc"=w524:i16[])
      n221 = invoke class="VI" method="Ctrl Val.Set (Deprecated)"(reference=w510, "Control Name"=w525, "Type Descriptor"=w524, "Flattened Data"=w519) -> ()  [unwired: 2 in, 6 out]
    }
    frame "setStringArray" {
      n222 = Unbundle By Name(w541) -> ("vi reference"=w543:refnum<vi>, "Controls formated"=w542:cluster{"name":string, "type desc":i16[]}[], "connID"=w540:refnum<k5>)
      n223 = TCP Read(connection ID=w540, bytes to read=4, error in (no error)=w549) -> (connection ID out=w565:refnum<k5>, data out=w564:string, error out=w567:errorcluster)  [unwired: 2 out]
      n224 = Type Cast(type=0, x=w564) -> (*(type *) &x=w563:i32)
      n225 = TCP Read(connection ID=w565, bytes to read=w563, error in (no error)=w567) -> (connection ID out=w562:refnum<k5>, data out=w556:string, error out=w561:errorcluster)  [unwired: 2 out]
      n226 = TCP Read(connection ID=w562, bytes to read=4, error in (no error)=w561) -> (connection ID out=w547:refnum<k5>, data out=w559:string, error out=w546:errorcluster)  [unwired: 2 out]
      n227 = call "deleteEndString.vi"("chars to delete"=5 ("y"), "string in"=w556) -> ("substring out"=w557:string)  [unwired: 9 out]
      n228 = Type Cast(type=0, x=w559) -> (*(type *) &x=w548:i32)
      n229 = for {
        N: w548 -> [_]
        tunnel: w547 -> [w578]
        tunnel: w546 -> [w577]
        tunnel: [w570] -> _
        tunnel: [w569] -> w545
        tunnel: [w568] -> w544 mode=indexing
        n230 = TCP Read(connection ID=w578, bytes to read=4, error in (no error)=w577) -> (connection ID out=w575:refnum<k5>, data out=w572:string, error out=w574:errorcluster)  [unwired: 2 out]
        n231 = Type Cast(type=0, x=w572) -> (*(type *) &x=w571:i32)
        n232 = TCP Read(connection ID=w575, bytes to read=w571, error in (no error)=w574) -> (connection ID out=w570:refnum<k5>, data out=w568:string, error out=w569:errorcluster)  [unwired: 2 out]
      }
      n233 = call "searchElement.vi"("input"=w542, "name"=w557) -> ("output"=w553:cluster{"name":string, "type desc":i16[]})  [unwired: 9 out]
      n234 = Variant To Flattened String(Variant=w544) -> (data string=w552:string)  [unwired: 1 out]
      n235 = Unbundle By Name(w553) -> ("name"=w555:string, "type desc"=w554:i16[])
      n236 = invoke class="VI" method="Ctrl Val.Set (Deprecated)"(reference=w543, "Control Name"=w555, "Type Descriptor"=w554, "Flattened Data"=w552) -> ()  [unwired: 2 in, 6 out]
    }
    frame "setFloatArray" {
      n237 = Unbundle By Name(w580) -> ("vi reference"=w582:refnum<vi>, "Controls formated"=w581:cluster{"name":string, "type desc":i16[]}[], "connID"=w579:refnum<k5>)
      n238 = TCP Read(connection ID=w579, bytes to read=4, error in (no error)=w583) -> (connection ID out=w609:refnum<k5>, data out=w608:string, error out=w611:errorcluster)  [unwired: 2 out]
      n239 = Type Cast(type=0, x=w608) -> (*(type *) &x=w607:i32)
      n240 = TCP Read(connection ID=w609, bytes to read=w607, error in (no error)=w611) -> (connection ID out=w606:refnum<k5>, data out=w598:string, error out=w605:errorcluster)  [unwired: 2 out]
      n241 = call "deleteEndString.vi"("chars to delete"=5 ("y"), "string in"=w598) -> ("substring out"=w599:string)  [unwired: 9 out]
      n242 = TCP Read(connection ID=w606, bytes to read=4, error in (no error)=w605) -> (connection ID out=w603:refnum<k5>, data out=w601:string, error out=w604:errorcluster)  [unwired: 2 out]
      n243 = Type Cast(type=0, x=w601) -> (*(type *) &x=w592:i32)
      n244 = Multiply(x=4, y=w592) -> (x*y=w594:i32)
      n245 = call "searchElement.vi"("input"=w581, "name"=w599) -> ("output"=w595:cluster{"name":string, "type desc":i16[]})  [unwired: 9 out]
      n246 = TCP Read(connection ID=w603, bytes to read=w594, error in (no error)=w604) -> (data out=w590:string, error out=w584:errorcluster)  [unwired: 3 out]
      n247 = Unflatten From String(type=sgl[] [], binary string=w590, data includes array or string size? (T)=FALSE) -> (value=w587:sgl[])  [unwired: 1 in, 3 out]
      n248 = Variant To Flattened String(Variant=w587) -> (data string=w591:string)  [unwired: 1 out]
      n249 = Unbundle By Name(w595) -> ("name"=w597:string, "type desc"=w596:i16[])
      n250 = invoke class="VI" method="Ctrl Val.Set (Deprecated)"(reference=w582, "Control Name"=w597, "Type Descriptor"=w596, "Flattened Data"=w591) -> ()  [unwired: 2 in, 6 out]
    }
    frame "setBooleanArray2D" {
      w636 = 4 ("bytes to read")
      n251 = Unbundle By Name(w613) -> ("vi reference"=w615:refnum<vi>, "Controls formated"=w614:cluster{"name":string, "type desc":i16[]}[], "connID"=w612:refnum<k5>)
      n252 = TCP Read(connection ID=w612, bytes to read=4, error in (no error)=w618) -> (connection ID out=w646:refnum<k5>, data out=w645:string, error out=w648:errorcluster)  [unwired: 2 out]
      n253 = Type Cast(type=0, x=w645) -> (*(type *) &x=w644:i32)
      n254 = TCP Read(connection ID=w646, bytes to read=w644, error in (no error)=w648) -> (connection ID out=w643:refnum<k5>, data out=w637:string, error out=w642:errorcluster)  [unwired: 2 out]
      n255 = call "deleteEndString.vi"("chars to delete"=5 ("y"), "string in"=w637) -> ("substring out"=w638:string)  [unwired: 9 out]
      n256 = TCP Read(connection ID=w643, bytes to read=w636, error in (no error)=w642) -> (connection ID out=w640:refnum<k5>, data out=w635:string, error out=w641:errorcluster)  [unwired: 2 out]
      n257 = Type Cast(type=0, x=w635) -> (*(type *) &x=w629:i32)
      n258 = TCP Read(connection ID=w640, bytes to read=w636, error in (no error)=w641) -> (connection ID out=w632:refnum<k5>, data out=w633:string, error out=w631:errorcluster)  [unwired: 2 out]
      n259 = call "searchElement.vi"("input"=w614, "name"=w638) -> ("output"=w625:cluster{"name":string, "type desc":i16[]})  [unwired: 9 out]
      n260 = Type Cast(type=0, x=w633) -> (*(type *) &x=w630:i32)
      n261 = Compound Arithmetic op=MULTIPLY(w629, w630, 1 ("value")) -> (w628:i32)
      n262 = TCP Read(connection ID=w632, bytes to read=w628, error in (no error)=w631) -> (data out=w623:string, error out=w617:errorcluster)  [unwired: 3 out]
      n263 = Unflatten From String(type=bool[][] [], binary string=w623, data includes array or string size? (T)=FALSE) -> (value=w622:bool[][])  [unwired: 1 in, 3 out]
      n264 = Variant To Flattened String(Variant=w622) -> (data string=w621:string)  [unwired: 1 out]
      n265 = Unbundle By Name(w625) -> ("name"=w627:string, "type desc"=w626:i16[])
      n266 = invoke class="VI" method="Ctrl Val.Set (Deprecated)"(reference=w615, "Control Name"=w627, "Type Descriptor"=w626, "Flattened Data"=w621) -> ()  [unwired: 2 in, 6 out]
    }
    frame "setIntArray2D" {
      w674 = 4 ("bytes to read")
      n267 = Unbundle By Name(w651) -> ("vi reference"=w653:refnum<vi>, "Controls formated"=w652:cluster{"name":string, "type desc":i16[]}[], "connID"=w650:refnum<k5>)
      n268 = TCP Read(connection ID=w650, bytes to read=4, error in (no error)=w656) -> (connection ID out=w684:refnum<k5>, data out=w683:string, error out=w686:errorcluster)  [unwired: 2 out]
      n269 = Type Cast(type=0, x=w683) -> (*(type *) &x=w682:i32)
      n270 = TCP Read(connection ID=w684, bytes to read=w682, error in (no error)=w686) -> (connection ID out=w681:refnum<k5>, data out=w675:string, error out=w680:errorcluster)  [unwired: 2 out]
      n271 = call "deleteEndString.vi"("chars to delete"=5 ("y"), "string in"=w675) -> ("substring out"=w676:string)  [unwired: 9 out]
      n272 = TCP Read(connection ID=w681, bytes to read=w674, error in (no error)=w680) -> (connection ID out=w678:refnum<k5>, data out=w673:string, error out=w679:errorcluster)  [unwired: 2 out]
      n273 = Type Cast(type=0, x=w673) -> (*(type *) &x=w667:i32)
      n274 = TCP Read(connection ID=w678, bytes to read=w674, error in (no error)=w679) -> (connection ID out=w670:refnum<k5>, data out=w671:string, error out=w669:errorcluster)  [unwired: 2 out]
      n275 = call "searchElement.vi"("input"=w652, "name"=w676) -> ("output"=w663:cluster{"name":string, "type desc":i16[]})  [unwired: 9 out]
      n276 = Type Cast(type=0, x=w671) -> (*(type *) &x=w668:i32)
      n277 = Compound Arithmetic op=MULTIPLY(w667, w668, 4 ("value")) -> (w666:i32)
      n278 = TCP Read(connection ID=w670, bytes to read=w666, error in (no error)=w669) -> (data out=w661:string, error out=w655:errorcluster)  [unwired: 3 out]
      n279 = Unflatten From String(type=i32[][] [], binary string=w661, data includes array or string size? (T)=FALSE) -> (value=w660:i32[][])  [unwired: 1 in, 3 out]
      n280 = Variant To Flattened String(Variant=w660) -> (data string=w659:string)  [unwired: 1 out]
      n281 = Unbundle By Name(w663) -> ("name"=w665:string, "type desc"=w664:i16[])
      n282 = invoke class="VI" method="Ctrl Val.Set (Deprecated)"(reference=w653, "Control Name"=w665, "Type Descriptor"=w664, "Flattened Data"=w659) -> ()  [unwired: 2 in, 6 out]
    }
    frame "setDoubleArray2D" {
      w712 = 4 ("bytes to read")
      n283 = Unbundle By Name(w689) -> ("vi reference"=w691:refnum<vi>, "Controls formated"=w690:cluster{"name":string, "type desc":i16[]}[], "connID"=w688:refnum<k5>)
      n284 = TCP Read(connection ID=w688, bytes to read=4, error in (no error)=w694) -> (connection ID out=w722:refnum<k5>, data out=w721:string, error out=w724:errorcluster)  [unwired: 2 out]
      n285 = Type Cast(type=0, x=w721) -> (*(type *) &x=w720:i32)
      n286 = TCP Read(connection ID=w722, bytes to read=w720, error in (no error)=w724) -> (connection ID out=w719:refnum<k5>, data out=w713:string, error out=w718:errorcluster)  [unwired: 2 out]
      n287 = call "deleteEndString.vi"("chars to delete"=5 ("y"), "string in"=w713) -> ("substring out"=w714:string)  [unwired: 9 out]
      n288 = TCP Read(connection ID=w719, bytes to read=w712, error in (no error)=w718) -> (connection ID out=w716:refnum<k5>, data out=w711:string, error out=w717:errorcluster)  [unwired: 2 out]
      n289 = Type Cast(type=0, x=w711) -> (*(type *) &x=w705:i32)
      n290 = TCP Read(connection ID=w716, bytes to read=w712, error in (no error)=w717) -> (connection ID out=w708:refnum<k5>, data out=w709:string, error out=w707:errorcluster)  [unwired: 2 out]
      n291 = call "searchElement.vi"("input"=w690, "name"=w714) -> ("output"=w701:cluster{"name":string, "type desc":i16[]})  [unwired: 9 out]
      n292 = Type Cast(type=0, x=w709) -> (*(type *) &x=w706:i32)
      n293 = Compound Arithmetic op=MULTIPLY(w705, w706, 8 ("value")) -> (w704:i32)
      n294 = TCP Read(connection ID=w708, bytes to read=w704, error in (no error)=w707) -> (data out=w699:string, error out=w693:errorcluster)  [unwired: 3 out]
      n295 = Unflatten From String(type=dbl[][] [], binary string=w699, data includes array or string size? (T)=FALSE) -> (value=w697:dbl[][])  [unwired: 1 in, 3 out]
      n296 = Variant To Flattened String(Variant=w697) -> (data string=w696:string)  [unwired: 1 out]
      n297 = Unbundle By Name(w701) -> ("name"=w703:string, "type desc"=w702:i16[])
      n298 = invoke class="VI" method="Ctrl Val.Set (Deprecated)"(reference=w691, "Control Name"=w703, "Type Descriptor"=w702, "Flattened Data"=w696) -> ()  [unwired: 2 in, 6 out]
    }
    frame "setStringArray2D" {
      w745 = 4 ("bytes to read")
      n299 = Unbundle By Name(w727) -> ("vi reference"=w729:refnum<vi>, "Controls formated"=w728:cluster{"name":string, "type desc":i16[]}[], "connID"=w726:refnum<k5>)
      n300 = TCP Read(connection ID=w726, bytes to read=4, error in (no error)=w736) -> (connection ID out=w755:refnum<k5>, data out=w754:string, error out=w757:errorcluster)  [unwired: 2 out]
      n301 = Type Cast(type=0, x=w754) -> (*(type *) &x=w753:i32)
      n302 = TCP Read(connection ID=w755, bytes to read=w753, error in (no error)=w757) -> (connection ID out=w752:refnum<k5>, data out=w746:string, error out=w751:errorcluster)  [unwired: 2 out]
      n303 = TCP Read(connection ID=w752, bytes to read=w745, error in (no error)=w751) -> (connection ID out=w749:refnum<k5>, data out=w744:string, error out=w750:errorcluster)  [unwired: 2 out]
      n304 = call "deleteEndString.vi"("chars to delete"=5 ("y"), "string in"=w746) -> ("substring out"=w747:string)  [unwired: 9 out]
      n305 = Type Cast(type=0, x=w744) -> (*(type *) &x=w735:i32)
      n306 = TCP Read(connection ID=w749, bytes to read=w745, error in (no error)=w750) -> (connection ID out=w733:refnum<k5>, data out=w742:string, error out=w732:errorcluster)  [unwired: 2 out]
      n307 = call "searchElement.vi"("input"=w728, "name"=w747) -> ("output"=w739:cluster{"name":string, "type desc":i16[]})  [unwired: 9 out]
      n308 = Type Cast(type=0, x=w742) -> (*(type *) &x=w734:i32)
      n309 = for {
        N: w735 -> [_]
        tunnel: w734 -> [w764]
        tunnel: w733 -> [w763]
        tunnel: w732 -> [w762]
        tunnel: [w761] -> _
        tunnel: [w760] -> w731
        tunnel: [w759] -> w730 mode=indexing
        n310 = for {
          N: w764 -> [_]
          tunnel: w763 -> [w774]
          tunnel: w762 -> [w773]
          tunnel: [w770] -> w761
          tunnel: [w769] -> w760
          tunnel: [w765] -> w759 mode=indexing
          n311 = TCP Read(connection ID=w774, error in (no error)=w773) -> (connection ID out=w772:refnum<k5>, data out=w767:string, error out=w771:errorcluster)  [unwired: 3 out]
          n312 = Type Cast(type=0, x=w767) -> (*(type *) &x=w766:i32)
          n313 = TCP Read(connection ID=w772, bytes to read=w766, error in (no error)=w771) -> (connection ID out=w770:refnum<k5>, data out=w765:string, error out=w769:errorcluster)  [unwired: 2 out]
        }
      }
      n314 = Variant To Flattened String(Variant=w730) -> (data string=w738:string)  [unwired: 1 out]
      n315 = Unbundle By Name(w739) -> ("name"=w741:string, "type desc"=w740:i16[])
      n316 = invoke class="VI" method="Ctrl Val.Set (Deprecated)"(reference=w729, "Control Name"=w741, "Type Descriptor"=w740, "Flattened Data"=w738) -> ()  [unwired: 2 in, 6 out]
    }
    frame "setFloatArray2D" {
      w799 = 4 ("bytes to read")
      n317 = Unbundle By Name(w776) -> ("vi reference"=w778:refnum<vi>, "Controls formated"=w777:cluster{"name":string, "type desc":i16[]}[], "connID"=w775:refnum<k5>)
      n318 = TCP Read(connection ID=w775, bytes to read=4, error in (no error)=w780) -> (connection ID out=w809:refnum<k5>, data out=w808:string, error out=w811:errorcluster)  [unwired: 2 out]
      n319 = Type Cast(type=0, x=w808) -> (*(type *) &x=w807:i32)
      n320 = TCP Read(connection ID=w809, bytes to read=w807, error in (no error)=w811) -> (connection ID out=w806:refnum<k5>, data out=w800:string, error out=w805:errorcluster)  [unwired: 2 out]
      n321 = call "deleteEndString.vi"("chars to delete"=5 ("y"), "string in"=w800) -> ("substring out"=w801:string)  [unwired: 9 out]
      n322 = TCP Read(connection ID=w806, bytes to read=w799, error in (no error)=w805) -> (connection ID out=w803:refnum<k5>, data out=w798:string, error out=w804:errorcluster)  [unwired: 2 out]
      n323 = Type Cast(type=0, x=w798) -> (*(type *) &x=w792:i32)
      n324 = TCP Read(connection ID=w803, bytes to read=w799, error in (no error)=w804) -> (connection ID out=w795:refnum<k5>, data out=w796:string, error out=w794:errorcluster)  [unwired: 2 out]
      n325 = call "searchElement.vi"("input"=w777, "name"=w801) -> ("output"=w788:cluster{"name":string, "type desc":i16[]})  [unwired: 9 out]
      n326 = Type Cast(type=0, x=w796) -> (*(type *) &x=w793:i32)
      n327 = Compound Arithmetic op=MULTIPLY(w792, w793, 4 ("value")) -> (w791:i32)
      n328 = TCP Read(connection ID=w795, bytes to read=w791, error in (no error)=w794) -> (data out=w786:string, error out=w779:errorcluster)  [unwired: 3 out]
      n329 = Unflatten From String(type=sgl[][] [], binary string=w786, data includes array or string size? (T)=FALSE) -> (value=w784:sgl[][])  [unwired: 1 in, 3 out]
      n330 = Variant To Flattened String(Variant=w784) -> (data string=w783:string)  [unwired: 1 out]
      n331 = Unbundle By Name(w788) -> ("name"=w790:string, "type desc"=w789:i16[])
      n332 = invoke class="VI" method="Ctrl Val.Set (Deprecated)"(reference=w778, "Control Name"=w790, "Type Descriptor"=w789, "Flattened Data"=w783) -> ()  [unwired: 2 in, 6 out]
    }
    frame "getBoolean" {
      n333 = Unbundle By Name(w816) -> ("vi reference"=w814:refnum<vi>, "Indicators formated"=w815:cluster{"name":string, "type desc":i16[]}[], "connID"=w813:refnum<k5>)
      n334 = TCP Read(connection ID=w813, bytes to read=4, error in (no error)=w823) -> (connection ID out=w827:refnum<k5>, data out=w830:string, error out=w826:errorcluster)  [unwired: 2 out]
      n335 = Type Cast(type=0, x=w830) -> (*(type *) &x=w828:i32)
      n336 = TCP Read(connection ID=w827, bytes to read=w828, error in (no error)=w826) -> (connection ID out=w821:refnum<k5>, data out=w825:string, error out=w820:errorcluster)  [unwired: 2 out]
      n337 = call "deleteEndString.vi"("chars to delete"=5, "string in"=w825) -> ("substring out"=w824:string)  [unwired: 9 out]
      n338 = call "searchElement.vi"("input"=w815, "name"=w824) -> ("output"=w832:cluster{"name":string, "type desc":i16[]})  [unwired: 9 out]
      n339 = Unbundle By Name(w832) -> ("name"=w831:string)
      n340 = invoke class="VI" method="Ctrl Val.Get (Deprecated)"(reference=w814, "Control Name"=w831) -> (error out=w817:errorcluster, "Get Control Value"=w818:string)  [unwired: 3 in, 3 out]
      n341 = TCP Write(connection ID=w821, data in=w818, error in (no error)=w820) -> (error out=w819:errorcluster)  [unwired: 3 out]
      n342 = call "setError.vi"("error"=w817) -> ()  [unwired: 1 out]
    }
    frame "getInt" {
      n343 = Unbundle By Name(w835) -> ("vi reference"=w837:refnum<vi>, "Indicators formated"=w836:cluster{"name":string, "type desc":i16[]}[], "connID"=w834:refnum<k5>)
      n344 = TCP Read(connection ID=w834, bytes to read=4, error in (no error)=w841) -> (connection ID out=w848:refnum<k5>, data out=w851:string, error out=w847:errorcluster)  [unwired: 2 out]
      n345 = Type Cast(type=0, x=w851) -> (*(type *) &x=w849:i32)
      n346 = TCP Read(connection ID=w848, bytes to read=w849, error in (no error)=w847) -> (connection ID out=w843:refnum<k5>, data out=w846:string, error out=w842:errorcluster)  [unwired: 2 out]
      n347 = call "deleteEndString.vi"("chars to delete"=5, "string in"=w846) -> ("substring out"=w845:string)  [unwired: 9 out]
      n348 = call "searchElement.vi"("input"=w836, "name"=w845) -> ("output"=w853:cluster{"name":string, "type desc":i16[]})  [unwired: 9 out]
      n349 = Unbundle By Name(w853) -> ("name"=w852:string)
      n350 = invoke class="VI" method="Ctrl Val.Get (Deprecated)"(reference=w837, "Control Name"=w852) -> (error out=w838:errorcluster, "Get Control Value"=w839:string)  [unwired: 3 in, 3 out]
      n351 = TCP Write(connection ID=w843, data in=w839, error in (no error)=w842) -> (error out=w840:errorcluster)  [unwired: 3 out]
      n352 = call "setError.vi"("error"=w838) -> ()  [unwired: 1 out]
    }
    frame "getDouble" {
      n353 = Unbundle By Name(w856) -> ("vi reference"=w858:refnum<vi>, "Indicators formated"=w857:cluster{"name":string, "type desc":i16[]}[], "connID"=w855:refnum<k5>)
      n354 = TCP Read(connection ID=w855, bytes to read=4, error in (no error)=w862) -> (connection ID out=w869:refnum<k5>, data out=w872:string, error out=w868:errorcluster)  [unwired: 2 out]
      n355 = Type Cast(type=0, x=w872) -> (*(type *) &x=w870:i32)
      n356 = TCP Read(connection ID=w869, bytes to read=w870, error in (no error)=w868) -> (connection ID out=w864:refnum<k5>, data out=w867:string, error out=w863:errorcluster)  [unwired: 2 out]
      n357 = call "deleteEndString.vi"("chars to delete"=5, "string in"=w867) -> ("substring out"=w866:string)  [unwired: 9 out]
      n358 = call "searchElement.vi"("input"=w857, "name"=w866) -> ("output"=w874:cluster{"name":string, "type desc":i16[]})  [unwired: 9 out]
      n359 = Unbundle By Name(w874) -> ("name"=w873:string)
      n360 = invoke class="VI" method="Ctrl Val.Get (Deprecated)"(reference=w858, "Control Name"=w873) -> (error out=w859:errorcluster, "Get Control Value"=w860:string)  [unwired: 3 in, 3 out]
      n361 = TCP Write(connection ID=w864, data in=w860, error in (no error)=w863) -> (error out=w861:errorcluster)  [unwired: 3 out]
      n362 = call "setError.vi"("error"=w859) -> ()  [unwired: 1 out]
    }
    frame "getString" {
      n363 = Unbundle By Name(w877) -> ("vi reference"=w879:refnum<vi>, "Indicators formated"=w878:cluster{"name":string, "type desc":i16[]}[], "connID"=w876:refnum<k5>)
      n364 = TCP Read(connection ID=w876, bytes to read=4, error in (no error)=w883) -> (connection ID out=w890:refnum<k5>, data out=w893:string, error out=w889:errorcluster)  [unwired: 2 out]
      n365 = Type Cast(type=0, x=w893) -> (*(type *) &x=w891:i32)
      n366 = TCP Read(connection ID=w890, bytes to read=w891, error in (no error)=w889) -> (connection ID out=w885:refnum<k5>, data out=w888:string, error out=w884:errorcluster)  [unwired: 2 out]
      n367 = call "deleteEndString.vi"("chars to delete"=5, "string in"=w888) -> ("substring out"=w887:string)  [unwired: 9 out]
      n368 = call "searchElement.vi"("input"=w878, "name"=w887) -> ("output"=w895:cluster{"name":string, "type desc":i16[]})  [unwired: 9 out]
      n369 = Unbundle By Name(w895) -> ("name"=w894:string)
      n370 = invoke class="VI" method="Ctrl Val.Get (Deprecated)"(reference=w879, "Control Name"=w894) -> (error out=w880:errorcluster, "Get Control Value"=w881:string)  [unwired: 3 in, 3 out]
      n371 = TCP Write(connection ID=w885, data in=w881, error in (no error)=w884) -> (error out=w882:errorcluster)  [unwired: 3 out]
      n372 = call "setError.vi"("error"=w880) -> ()  [unwired: 1 out]
    }
    frame "getFloat" {
      n373 = Unbundle By Name(w900) -> ("vi reference"=w899:refnum<vi>, "Indicators formated"=w898:cluster{"name":string, "type desc":i16[]}[], "connID"=w897:refnum<k5>)
      n374 = TCP Read(connection ID=w897, bytes to read=4, error in (no error)=w903) -> (connection ID out=w911:refnum<k5>, data out=w914:string, error out=w910:errorcluster)  [unwired: 2 out]
      n375 = Type Cast(type=0, x=w914) -> (*(type *) &x=w912:i32)
      n376 = TCP Read(connection ID=w911, bytes to read=w912, error in (no error)=w910) -> (connection ID out=w906:refnum<k5>, data out=w909:string, error out=w905:errorcluster)  [unwired: 2 out]
      n377 = call "deleteEndString.vi"("chars to delete"=5, "string in"=w909) -> ("substring out"=w908:string)  [unwired: 9 out]
      n378 = call "searchElement.vi"("input"=w898, "name"=w908) -> ("output"=w916:cluster{"name":string, "type desc":i16[]})  [unwired: 9 out]
      n379 = Unbundle By Name(w916) -> ("name"=w915:string)
      n380 = invoke class="VI" method="Ctrl Val.Get (Deprecated)"(reference=w899, "Control Name"=w915) -> (error out=w901:errorcluster, "Get Control Value"=w904:string)  [unwired: 3 in, 3 out]
      n381 = TCP Write(connection ID=w906, data in=w904, error in (no error)=w905) -> (error out=w902:errorcluster)  [unwired: 3 out]
      n382 = call "setError.vi"("error"=w901) -> ()  [unwired: 1 out]
    }
    frame "getBooleanArray" {
      n383 = Unbundle By Name(w919) -> ("vi reference"=w921:refnum<vi>, "Indicators formated"=w920:cluster{"name":string, "type desc":i16[]}[], "connID"=w918:refnum<k5>)
      n384 = TCP Read(connection ID=w918, bytes to read=4, error in (no error)=w925) -> (connection ID out=w932:refnum<k5>, data out=w935:string, error out=w931:errorcluster)  [unwired: 2 out]
      n385 = Type Cast(type=0, x=w935) -> (*(type *) &x=w933:i32)
      n386 = TCP Read(connection ID=w932, bytes to read=w933, error in (no error)=w931) -> (connection ID out=w927:refnum<k5>, data out=w930:string, error out=w926:errorcluster)  [unwired: 2 out]
      n387 = call "deleteEndString.vi"("chars to delete"=5, "string in"=w930) -> ("substring out"=w929:string)  [unwired: 9 out]
      n388 = call "searchElement.vi"("input"=w920, "name"=w929) -> ("output"=w937:cluster{"name":string, "type desc":i16[]})  [unwired: 9 out]
      n389 = Unbundle By Name(w937) -> ("name"=w936:string)
      n390 = invoke class="VI" method="Ctrl Val.Get (Deprecated)"(reference=w921, "Control Name"=w936) -> (error out=w922:errorcluster, "Get Control Value"=w923:string)  [unwired: 3 in, 3 out]
      n391 = TCP Write(connection ID=w927, data in=w923, error in (no error)=w926) -> (error out=w924:errorcluster)  [unwired: 3 out]
      n392 = call "setError.vi"("error"=w922) -> ()  [unwired: 1 out]
    }
    frame "getIntArray" {
      n393 = Unbundle By Name(w942) -> ("vi reference"=w941:refnum<vi>, "Indicators formated"=w940:cluster{"name":string, "type desc":i16[]}[], "connID"=w939:refnum<k5>)
      n394 = TCP Read(connection ID=w939, bytes to read=4, error in (no error)=w946) -> (connection ID out=w953:refnum<k5>, data out=w956:string, error out=w952:errorcluster)  [unwired: 2 out]
      n395 = Type Cast(type=0, x=w956) -> (*(type *) &x=w954:i32)
      n396 = TCP Read(connection ID=w953, bytes to read=w954, error in (no error)=w952) -> (connection ID out=w948:refnum<k5>, data out=w951:string, error out=w947:errorcluster)  [unwired: 2 out]
      n397 = call "deleteEndString.vi"("chars to delete"=5, "string in"=w951) -> ("substring out"=w950:string)  [unwired: 9 out]
      n398 = call "searchElement.vi"("input"=w940, "name"=w950) -> ("output"=w958:cluster{"name":string, "type desc":i16[]})  [unwired: 9 out]
      n399 = Unbundle By Name(w958) -> ("name"=w957:string)
      n400 = invoke class="VI" method="Ctrl Val.Get (Deprecated)"(reference=w941, "Control Name"=w957) -> (error out=w943:errorcluster, "Get Control Value"=w944:string)  [unwired: 3 in, 3 out]
      n401 = TCP Write(connection ID=w948, data in=w944, error in (no error)=w947) -> (error out=w945:errorcluster)  [unwired: 3 out]
      n402 = call "setError.vi"("error"=w943) -> ()  [unwired: 1 out]
    }
    frame "getDoubleArray" {
      n403 = Unbundle By Name(w962) -> ("vi reference"=w963:refnum<vi>, "Indicators formated"=w961:cluster{"name":string, "type desc":i16[]}[], "connID"=w960:refnum<k5>)
      n404 = TCP Read(connection ID=w960, bytes to read=4, error in (no error)=w967) -> (connection ID out=w974:refnum<k5>, data out=w977:string, error out=w973:errorcluster)  [unwired: 2 out]
      n405 = Type Cast(type=0, x=w977) -> (*(type *) &x=w975:i32)
      n406 = TCP Read(connection ID=w974, bytes to read=w975, error in (no error)=w973) -> (connection ID out=w969:refnum<k5>, data out=w972:string, error out=w968:errorcluster)  [unwired: 2 out]
      n407 = call "deleteEndString.vi"("chars to delete"=5, "string in"=w972) -> ("substring out"=w971:string)  [unwired: 9 out]
      n408 = call "searchElement.vi"("input"=w961, "name"=w971) -> ("output"=w979:cluster{"name":string, "type desc":i16[]})  [unwired: 9 out]
      n409 = Unbundle By Name(w979) -> ("name"=w978:string)
      n410 = invoke class="VI" method="Ctrl Val.Get (Deprecated)"(reference=w963, "Control Name"=w978) -> (error out=w964:errorcluster, "Get Control Value"=w965:string)  [unwired: 3 in, 3 out]
      n411 = TCP Write(connection ID=w969, data in=w965, error in (no error)=w968) -> (error out=w966:errorcluster)  [unwired: 3 out]
      n412 = call "setError.vi"("error"=w964) -> ()  [unwired: 1 out]
    }
    frame "getStringArray" {
      n413 = Unbundle By Name(w982) -> ("vi reference"=w983:refnum<vi>, "Indicators formated"=w984:cluster{"name":string, "type desc":i16[]}[], "connID"=w981:refnum<k5>)
      n414 = TCP Read(connection ID=w981, bytes to read=4, error in (no error)=w988) -> (connection ID out=w995:refnum<k5>, data out=w998:string, error out=w994:errorcluster)  [unwired: 2 out]
      n415 = Type Cast(type=0, x=w998) -> (*(type *) &x=w996:i32)
      n416 = TCP Read(connection ID=w995, bytes to read=w996, error in (no error)=w994) -> (connection ID out=w990:refnum<k5>, data out=w993:string, error out=w989:errorcluster)  [unwired: 2 out]
      n417 = call "deleteEndString.vi"("chars to delete"=5, "string in"=w993) -> ("substring out"=w992:string)  [unwired: 9 out]
      n418 = call "searchElement.vi"("input"=w984, "name"=w992) -> ("output"=w1000:cluster{"name":string, "type desc":i16[]})  [unwired: 9 out]
      n419 = Unbundle By Name(w1000) -> ("name"=w999:string)
      n420 = invoke class="VI" method="Ctrl Val.Get (Deprecated)"(reference=w983, "Control Name"=w999) -> (error out=w985:errorcluster, "Get Control Value"=w986:string)  [unwired: 3 in, 3 out]
      n421 = TCP Write(connection ID=w990, data in=w986, error in (no error)=w989) -> (error out=w987:errorcluster)  [unwired: 3 out]
      n422 = call "setError.vi"("error"=w985) -> ()  [unwired: 1 out]
    }
    frame "getFloatArray" {
      # "creo que aquí había un error \ntomabas controls formated y \ncreo que son los inidcators"
      n423 = Unbundle By Name(w1003) -> ("vi reference"=w1005:refnum<vi>, "Indicators formated"=w1004:cluster{"name":string, "type desc":i16[]}[], "connID"=w1002:refnum<k5>)
      n424 = TCP Read(connection ID=w1002, bytes to read=4, error in (no error)=w1008) -> (connection ID out=w1016:refnum<k5>, data out=w1019:string, error out=w1015:errorcluster)  [unwired: 2 out]
      n425 = Type Cast(type=0, x=w1019) -> (*(type *) &x=w1017:i32)
      n426 = TCP Read(connection ID=w1016, bytes to read=w1017, error in (no error)=w1015) -> (connection ID out=w1011:refnum<k5>, data out=w1014:string, error out=w1010:errorcluster)  [unwired: 2 out]
      n427 = call "deleteEndString.vi"("chars to delete"=5, "string in"=w1014) -> ("substring out"=w1013:string)  [unwired: 9 out]
      n428 = call "searchElement.vi"("input"=w1004, "name"=w1013) -> ("output"=w1021:cluster{"name":string, "type desc":i16[]})  [unwired: 9 out]
      n429 = Unbundle By Name(w1021) -> ("name"=w1020:string)
      n430 = invoke class="VI" method="Ctrl Val.Get (Deprecated)"(reference=w1005, "Control Name"=w1020) -> (error out=w1006:errorcluster, "Get Control Value"=w1009:string)  [unwired: 3 in, 3 out]
      n431 = TCP Write(connection ID=w1011, data in=w1009, error in (no error)=w1010) -> (error out=w1007:errorcluster)  [unwired: 3 out]
      n432 = call "setError.vi"("error"=w1006) -> ()  [unwired: 1 out]
    }
    frame "getBooleanArray2D" {
      n433 = Unbundle By Name(w1026) -> ("vi reference"=w1025:refnum<vi>, "Indicators formated"=w1024:cluster{"name":string, "type desc":i16[]}[], "connID"=w1023:refnum<k5>)
      n434 = TCP Read(connection ID=w1023, bytes to read=4, error in (no error)=w1030) -> (connection ID out=w1037:refnum<k5>, data out=w1040:string, error out=w1036:errorcluster)  [unwired: 2 out]
      n435 = Type Cast(type=0, x=w1040) -> (*(type *) &x=w1038:i32)
      n436 = TCP Read(connection ID=w1037, bytes to read=w1038, error in (no error)=w1036) -> (connection ID out=w1032:refnum<k5>, data out=w1035:string, error out=w1031:errorcluster)  [unwired: 2 out]
      n437 = call "deleteEndString.vi"("chars to delete"=5, "string in"=w1035) -> ("substring out"=w1034:string)  [unwired: 9 out]
      n438 = call "searchElement.vi"("input"=w1024, "name"=w1034) -> ("output"=w1042:cluster{"name":string, "type desc":i16[]})  [unwired: 9 out]
      n439 = Unbundle By Name(w1042) -> ("name"=w1041:string)
      n440 = invoke class="VI" method="Ctrl Val.Get (Deprecated)"(reference=w1025, "Control Name"=w1041) -> (error out=w1027:errorcluster, "Get Control Value"=w1028:string)  [unwired: 3 in, 3 out]
      n441 = TCP Write(connection ID=w1032, data in=w1028, error in (no error)=w1031) -> (error out=w1029:errorcluster)  [unwired: 3 out]
      n442 = call "setError.vi"("error"=w1027) -> ()  [unwired: 1 out]
    }
    frame "getIntArray2D" {
      n443 = Unbundle By Name(w1045) -> ("vi reference"=w1047:refnum<vi>, "Indicators formated"=w1046:cluster{"name":string, "type desc":i16[]}[], "connID"=w1044:refnum<k5>)
      n444 = TCP Read(connection ID=w1044, bytes to read=4, error in (no error)=w1051) -> (connection ID out=w1058:refnum<k5>, data out=w1061:string, error out=w1057:errorcluster)  [unwired: 2 out]
      n445 = Type Cast(type=0, x=w1061) -> (*(type *) &x=w1059:i32)
      n446 = TCP Read(connection ID=w1058, bytes to read=w1059, error in (no error)=w1057) -> (connection ID out=w1053:refnum<k5>, data out=w1056:string, error out=w1052:errorcluster)  [unwired: 2 out]
      n447 = call "deleteEndString.vi"("chars to delete"=5, "string in"=w1056) -> ("substring out"=w1055:string)  [unwired: 9 out]
      n448 = call "searchElement.vi"("input"=w1046, "name"=w1055) -> ("output"=w1063:cluster{"name":string, "type desc":i16[]})  [unwired: 9 out]
      n449 = Unbundle By Name(w1063) -> ("name"=w1062:string)
      n450 = invoke class="VI" method="Ctrl Val.Get (Deprecated)"(reference=w1047, "Control Name"=w1062) -> (error out=w1048:errorcluster, "Get Control Value"=w1049:string)  [unwired: 3 in, 3 out]
      n451 = TCP Write(connection ID=w1053, data in=w1049, error in (no error)=w1052) -> (error out=w1050:errorcluster)  [unwired: 3 out]
      n452 = call "setError.vi"("error"=w1048) -> ()  [unwired: 1 out]
    }
    frame "getDoubleArray2D" {
      n453 = Unbundle By Name(w1066) -> ("vi reference"=w1068:refnum<vi>, "Indicators formated"=w1067:cluster{"name":string, "type desc":i16[]}[], "connID"=w1065:refnum<k5>)
      n454 = TCP Read(connection ID=w1065, bytes to read=4, error in (no error)=w1072) -> (connection ID out=w1079:refnum<k5>, data out=w1082:string, error out=w1078:errorcluster)  [unwired: 2 out]
      n455 = Type Cast(type=0, x=w1082) -> (*(type *) &x=w1080:i32)
      n456 = TCP Read(connection ID=w1079, bytes to read=w1080, error in (no error)=w1078) -> (connection ID out=w1074:refnum<k5>, data out=w1077:string, error out=w1073:errorcluster)  [unwired: 2 out]
      n457 = call "deleteEndString.vi"("chars to delete"=5, "string in"=w1077) -> ("substring out"=w1076:string)  [unwired: 9 out]
      n458 = call "searchElement.vi"("input"=w1067, "name"=w1076) -> ("output"=w1084:cluster{"name":string, "type desc":i16[]})  [unwired: 9 out]
      n459 = Unbundle By Name(w1084) -> ("name"=w1083:string)
      n460 = invoke class="VI" method="Ctrl Val.Get (Deprecated)"(reference=w1068, "Control Name"=w1083) -> (error out=w1069:errorcluster, "Get Control Value"=w1070:string)  [unwired: 3 in, 3 out]
      n461 = TCP Write(connection ID=w1074, data in=w1070, error in (no error)=w1073) -> (error out=w1071:errorcluster)  [unwired: 3 out]
      n462 = call "setError.vi"("error"=w1069) -> ()  [unwired: 1 out]
    }
    frame "getStringArray2D" {
      n463 = Unbundle By Name(w1087) -> ("vi reference"=w1089:refnum<vi>, "Indicators formated"=w1088:cluster{"name":string, "type desc":i16[]}[], "connID"=w1086:refnum<k5>)
      n464 = TCP Read(connection ID=w1086, bytes to read=4, error in (no error)=w1091) -> (connection ID out=w1100:refnum<k5>, data out=w1103:string, error out=w1099:errorcluster)  [unwired: 2 out]
      n465 = Type Cast(type=0, x=w1103) -> (*(type *) &x=w1101:i32)
      n466 = TCP Read(connection ID=w1100, bytes to read=w1101, error in (no error)=w1099) -> (connection ID out=w1095:refnum<k5>, data out=w1098:string, error out=w1094:errorcluster)  [unwired: 2 out]
      n467 = call "deleteEndString.vi"("chars to delete"=5, "string in"=w1098) -> ("substring out"=w1097:string)  [unwired: 9 out]
      n468 = call "searchElement.vi"("input"=w1088, "name"=w1097) -> ("output"=w1105:cluster{"name":string, "type desc":i16[]})  [unwired: 9 out]
      n469 = Unbundle By Name(w1105) -> ("name"=w1104:string)
      n470 = invoke class="VI" method="Ctrl Val.Get (Deprecated)"(reference=w1089, "Control Name"=w1104) -> (error out=w1090:errorcluster, "Get Control Value"=w1093:string)  [unwired: 3 in, 3 out]
      n471 = TCP Write(connection ID=w1095, data in=w1093, error in (no error)=w1094) -> (error out=w1092:errorcluster)  [unwired: 3 out]
      n472 = call "setError.vi"("error"=w1090) -> ()  [unwired: 1 out]
    }
    frame "getFloatArray2D" {
      n473 = Unbundle By Name(w1109) -> ("vi reference"=w1110:refnum<vi>, "Indicators formated"=w1108:cluster{"name":string, "type desc":i16[]}[], "connID"=w1107:refnum<k5>)
      n474 = TCP Read(connection ID=w1107, bytes to read=4, error in (no error)=w1113) -> (connection ID out=w1121:refnum<k5>, data out=w1124:string, error out=w1120:errorcluster)  [unwired: 2 out]
      n475 = Type Cast(type=0, x=w1124) -> (*(type *) &x=w1122:i32)
      n476 = TCP Read(connection ID=w1121, bytes to read=w1122, error in (no error)=w1120) -> (connection ID out=w1116:refnum<k5>, data out=w1119:string, error out=w1115:errorcluster)  [unwired: 2 out]
      n477 = call "deleteEndString.vi"("chars to delete"=5, "string in"=w1119) -> ("substring out"=w1118:string)  [unwired: 9 out]
      n478 = call "searchElement.vi"("input"=w1108, "name"=w1118) -> ("output"=w1126:cluster{"name":string, "type desc":i16[]})  [unwired: 9 out]
      n479 = Unbundle By Name(w1126) -> ("name"=w1125:string)
      n480 = invoke class="VI" method="Ctrl Val.Get (Deprecated)"(reference=w1110, "Control Name"=w1125) -> (error out=w1111:errorcluster, "Get Control Value"=w1114:string)  [unwired: 3 in, 3 out]
      n481 = TCP Write(connection ID=w1116, data in=w1114, error in (no error)=w1115) -> (error out=w1112:errorcluster)  [unwired: 3 out]
      n482 = call "setError.vi"("error"=w1111) -> ()  [unwired: 1 out]
    }
  }
  "ParserStateOUT" <- w5
  "error out" <- w4
